vi "CPP-Multiplot.vi"(1 "Job Directory":path) -> (2 "Saved Automatically?":bool, 3 "gnuplotScript":string, 4 "Plot data file":path)   [LabVIEW 2022 SP3]
uses:
  gnuplotScriptComponents/plotstyle.ctl
  gnuplotScriptComponents/graphPeripherals.ctl
  gnuplotScriptComponents/minAndMax.ctl
  gnuplotScriptComponents/AutoManualNumber.ctl
  gnuplotScriptComponents/ticsAndGrids.ctl
  gnuplotScriptComponents/tics.ctl
  gnuplotScriptComponents/grids.ctl
  gnuplotScriptComponents/legendProperties.ctl
  gnuplotScriptComponents/legendAppearance.ctl
  gnuplotScriptComponents/alignment.ctl
  gnuplotScriptComponents/at.ctl
  gnuplotScriptComponents/margins.ctl
  gnuplotScriptComponents/source.ctl
  gnuplotScriptComponents/Master_Legend.ctl
  gnuplotScriptComponents/MasterPeripherals.ctl
  Error bar Type.ctl
  gnuplotScriptComponents/axisName.ctl
  Results_plotter_Global.vi
  Data plotting/subVIs/Plot_Values_Global.vi
panel:
  out "Multi_Plot":bool
  in  "OpenLogfile?":bool
  in  "Show Script Editor?":bool
  in  "Tab Control":T1(tab)=enum."Appearance"
  in  "setupPath":path
  in  "saveMPsetup":bool
  in  "loadMPsetup":bool
  in  "Each Graph contains:":T2=enum."Series"
  in  "Rows from:":T2=enum."Until done"
  in  "Columns from:":T2=enum."Yellow Filter"
  in  "Margins":T3={"Top"=2.0, "Bottom"=2.0, "Left"=2.0, "Right"=2.0}
  in  "Height (in)":dbl=7.0 min=0.5 step=0.5 format="%.1f"
  in  "Width (in)":dbl=10.0 min=0.5 step=0.5 format="%.1f"
  in  "nRows":u8=3 min=1
  in  "nCols":u8=3 min=1
  in  "ScaleAdjust":dbl=0.9 min=0.1 max=2.0 step=0.1
  in  "Swop Series and Plots":bool
  in  "PlotTitlesNeed $$?":bool=TRUE
  in  "Show Channels with range of Values?":bool
  in  "ManualPlotTitles":string[](array[string])
  out "AutoPlotTitles":string[](array[string])
  in  "Individual Plot Titles":bool=TRUE
  in  "Page Title Pre Block":string
  in  "Page Title Post Block":string
  in  "Values to include in Page Title":i32[](listbox)
  in  "Plot Title Offset (characters)":cluster{"horizontal":dbl, "vertical":dbl}
  out "Final Title":string
  in  "PlotNamesNeed $$?":bool=TRUE
  in  "Plot Legends Manual":string[](array[string])
  in  "Plotstyles":T4[](array[typedef])=[{"Style"="linespoints", "Color"=16711680, "PointType"=1, "PointSize"=1.0, "LineWidth"=1.0, "LineType"=1}, {"Style"="linespoints", "Color"=16860, "PointType"=2, "PointSize"=1.0, "LineWidth"=1.0, "LineType"=1}, {"Style"="linespoints", "Color"=51228, "PointType"=3, "PointSize"=1.0, "LineWidth"=1.0, "LineType"=1}, {"Style"="linespoints", "Color"=0, "PointType"=4, "PointSize"=1.0, "LineWidth"=1.0, "LineType"=1}, {"Style"="linespoints", "Color"=9567230, "PointType"=5, "PointSize"=1.0, "LineWidth"=1.0, "LineType"=1}, {"Style"="linespoints", "Color"=12369084, "PointType"=6, "PointSize"=1.0, "LineWidth"=1.0, "LineType"=1}, {"Style"="linespoints", "Color"=15667967, "PointType"=7, "PointSize"=1.0, "LineWidth"=1.0, "LineType"=1}, {"Style"="linespoints", "Color"=15400704, "PointType"=8, "PointSize"=1.0, "LineWidth"=1.0, "LineType"=1}, {"Style"="linespoints", "Color"=128, "PointType"=9, "PointSize"=1.0, "LineWidth"=1.0, "LineType"=1}, {"Style"="linespoints", "Color"=8404992, "PointType"=10, "PointSize"=1.0, "LineWidth"=1.0, "LineType"=1}, {"Style"="linespoints", "Color"=6737151, "PointType"=11, "PointSize"=1.0, "LineWidth"=1.0, "LineType"=1}, {"Style"="linespoints", "Color"=8388672, "PointType"=12, "PointSize"=1.0, "LineWidth"=1.0, "LineType"=1}, {"Style"="linespoints", "Color"=16740303, "PointType"=13, "PointSize"=1.0, "LineWidth"=1.0, "LineType"=1}, {"Style"="linespoints", "Color"=16764006, "PointType"=14, "PointSize"=1.0, "LineWidth"=1.0, "LineType"=1}, {"Style"="linespoints", "Color"=8421376, "PointType"=15, "PointSize"=1.0, "LineWidth"=1.0, "LineType"=1}, {"Style"="linespoints", "Color"=65408, "PointType"=16, "PointSize"=1.0, "LineWidth"=1.0, "LineType"=1}] caption="Style                              Colour  PointType    PointSize     Linewidth      Linestyle" {"LineType" min=1 max=6 step=1; "LineWidth" min=1 max=6 step=1; "PointSize" min=0 step=0.1}
  out "Plot Legends Auto":string[](array[string])
  out "No of Series supplied":i32
  out "No of Graph Slots Available":i32
  in  "Plot Legends":bool=TRUE
  in  "Error Bar Type":T5=enum."Standard Error"
  in  "X axis label":enum32{"Autolabel", "Manual Label"}(tab)
  out "X or theta label":string
  in  "X or theta label Manual":string
  in  "LegendProperties":T6={"Appearance"={"layout"="", "text-sample order"="", "key order"="", "surroundingBox"="", "MaxRows"=0, "MaxCols"=0, "WidthAdjust"=0.0}, "Alignment"={"Horizontal"="", "Vertical"=""}, "Location"="auto", "\"At\" location"={"XcoordSys"="", "YcoordSys"="", "Xvalue"=0.0, "Yvalue"=0.0}}
  in  "Y/R tics And Grids":T10={"tics"={"ticMin"=0.0, "ticStep"=5.0, "ticMax"=0.0, "minorDivsPerMajor"=2, "ticSpacing"=enum."Approx n Tics (rounded)", "ticPosition"=enum."Inside, no mirror"}, "Grids"={"Gridlines"=enum."No grids", "Zeroaxis"=enum."No zero axis"}, "Mapping"=enum."Lin"}
  in  "X/Theta tics And Grids":T10={"tics"={"ticMin"=0.0, "ticStep"=5.0, "ticMax"=0.0, "minorDivsPerMajor"=2, "ticSpacing"=enum."Approx n Tics (rounded)", "ticPosition"=enum."Inside, no mirror"}, "Grids"={"Gridlines"=enum."Major grid", "Zeroaxis"=enum."No zero axis"}, "Mapping"=enum."Lin"}
  in  "PlotType":enum32{"XY", "Polar", "Time"}(tab)
  in  "yAxisBounds":T13={"Min"={"Auto"=TRUE, "Value"=0.0}, "Max"={"Auto"=TRUE, "Value"=0.0}}
  in  "Additional XYgnuplot":string
  in  "xAxisBounds":T13={"Min"={"Auto"=TRUE, "Value"=0.0}, "Max"={"Auto"=TRUE, "Value"=0.0}}
  in  "Set bounds using XY Plot \non Results file plotter":bool
  in  "Angle Units":bool=TRUE
  in  "AngleMode":string(combo)="Compass"
  in  "wrapGapsUpTo:":dbl=30.0 step=0.1
  in  "Additional Polar gnuplot":string
  in  "rAxisBounds":T13={"Min"={"Auto"=FALSE, "Value"=0.0}, "Max"={"Auto"=FALSE, "Value"=1.5}}
  out "Time format?":bool
  in  "Time/Date Format":string(combo)="%I:%M %p\\n%d-%b-%y"
  in  "Select Time Zone":u32(ring)=142 items=["Abbreviation (Time Zone Name)", "A (Alpha Time Zone)", "ACDT (Australian Central Daylight Time  CDT ÇƒÏ Central Daylight Time CDST ÇƒÏ Central Daylight Savings Time)", "ACST (Australian Central Standard Time  CST ÇƒÏ Central Standard Time)", "ACT (Acre Time)", "ACT (Australian Central Time)", "ACWST (Australian Central Western Standard Time)", "ADT (Arabia Daylight Time  AST ÇƒÏ Arabia Summer Time)", "ADT (Atlantic Daylight Time  ADST ÇƒÏ Atlantic Daylight Saving Time AST ÇƒÏ Atlantic Summer Time  HAA ÇƒÏ Heure Avancv©e de l'Atlantique (French))", "AEDT (Australian Eastern Daylight Time  EDT ÇƒÏ Eastern Daylight Time EDST ÇƒÏ Eastern Daylight Saving Time)", "AEST (Australian Eastern Standard Time  EST ÇƒÏ Eastern Standard Time AET ÇƒÏ Australian Eastern Time)", "AET (Australian Eastern Time)", "AFT (Afghanistan Time)", "AKDT (Alaska Daylight Time  ADST ÇƒÏ Alaska Daylight Saving Time)", "AKST (Alaska Standard Time  AT ÇƒÏ Alaska Time)", "ALMT (Alma-Ata Time)", "AMST (Amazon Summer Time)", "AMST (Armenia Summer Time  AMDT ÇƒÏ Armenia Daylight Time)", "AMT (Amazon Time)", "AMT (Armenia Time)", "ANAST (Anadyr Summer Time)", "ANAT (Anadyr Time)", "AQTT (Aqtobe Time)", "ART (Argentina Time)", "AST (Arabia Standard Time  AST ÇƒÏ Arabic Standard Time AST ÇƒÏ Al Manamah Standard Time)", "AST (Atlantic Standard Time  AT ÇƒÏ Atlantic Time  AST ÇƒÏ Tiempo Estv∞ndar del Atlv∞ntico (Spanish) HNA ÇƒÏ Heure Normale de l'Atlantique (French))", "AT (Atlantic Time)", "AWDT (Australian Western Daylight Time  WDT ÇƒÏ Western Daylight Time WST ÇƒÏ Western Summer Time)", "AWST (Australian Western Standard Time  WST ÇƒÏ Western Standard Time WAT ÇƒÏ Western Australia Time)", "AZOST (Azores Summer Time  AZODT ÇƒÏ Azores Daylight Time)", "AZOT (Azores Time  AZOST ÇƒÏ Azores Standard Time)", "AZST (Azerbaijan Summer Time)", "AZT (Azerbaijan Time)", "AoE (Anywhere on Earth)", "B (Bravo Time Zone)", "BNT (Brunei Darussalam Time  BDT ÇƒÏ Brunei Time)", "BOT (Bolivia Time)", "BRST (Brasv?lia Summer Time  BST ÇƒÏ Brazil Summer Time BST ÇƒÏ Brazilian Summer Time)", "BRT (Brasv?lia Time  BT ÇƒÏ Brazil Time BT ÇƒÏ Brazilian Time)", "BST (Bangladesh Standard Time)", "BST (Bougainville Standard Time)", "BST (British Summer Time  BDT ÇƒÏ British Daylight Time BDST ÇƒÏ British Daylight Saving Time)", "BTT (Bhutan Time)", "C (Charlie Time Zone)", "CAST (Casey Time)", "CAT (Central Africa Time)", "CCT (Cocos Islands Time)", "CDT (Central Daylight Time  CDST ÇƒÏ Central Daylight Saving Time NACDT ÇƒÏ North American Central Daylight Time  HAC ÇƒÏ Heure Avancv©e du Centre (French))", "CDT (Cuba Daylight Time)", "CEST (Central European Summer Time  CEDT ÇƒÏ Central European Daylight Time ECST ÇƒÏ European Central Summer Time  MESZ ÇƒÏ Mitteleuropvßische Sommerzeit (German))", "CET (Central European Time  ECT ÇƒÏ European Central Time CET ÇƒÏ Central Europe Time  MEZ ÇƒÏ Mitteleuropvßische Zeit (German))", "CHADT (Chatham Island Daylight Time  CDT ÇƒÏ Chatham Daylight Time)", "CHAST (Chatham Island Standard Time)", "CHOST (Choibalsan Summer Time  CHODT ÇƒÏ Choibalsan Daylight Time CHODST ÇƒÏ Choibalsan Daylight Saving Time)", "CHOST (Choibalsan Summer Time)", "CHOT (Choibalsan Time)", "CHUT (Chuuk Time)", "CIDST (Cayman Islands Daylight Saving Time)", "CIST (Cayman Islands Standard Time  CIT ÇƒÏ Cayman Islands Time)", "CKT (Cook Island Time)", "CLST (Chile Summer Time  CLDT ÇƒÏ Chile Daylight Time)", "CLT (Chile Standard Time  CT ÇƒÏ Chile Time CLST ÇƒÏ Chile Standard Time)", "COT (Colombia Time)", "CST (Central Standard Time  CT ÇƒÏ Central Time NACST ÇƒÏ North American Central Standard Time  CST ÇƒÏ Tiempo Central Estv∞ndar (Spanish) HNC ÇƒÏ Heure Normale du Centre (French))", "CST (China Standard Time)", "CST (Cuba Standard Time)", "CT (Central Time)", "CVT (Cape Verde Time)", "CXT (Christmas Island Time)", "ChST (Chamorro Standard Time  GST ÇƒÏ Guam Standard Time)", "D (Delta Time Zone)", "DAVT (Davis Time)", "DDUT (Dumont-d'Urville Time)", "E (Echo Time Zone)", "EASST (Easter Island Summer Time  EADT ÇƒÏ Easter Island Daylight Time)", "EAST (Easter Island Standard Time)", "EAT (Eastern Africa Time  EAT ÇƒÏ East Africa Time)", "ECT (Ecuador Time)", "EDT (Eastern Daylight Time  EDST ÇƒÏ Eastern Daylight Savings Time NAEDT ÇƒÏ North American Eastern Daylight Time  HAE ÇƒÏ Heure Avancv©e de l'Est (French) EDT ÇƒÏ Tiempo de verano del Este (Spanish))", "EEST (Eastern European Summer Time  EEDT ÇƒÏ Eastern European Daylight Time  OESZ ÇƒÏ Osteuropvßische Sommerzeit (German))", "EET (Eastern European Time  OEZ ÇƒÏ Osteuropvßische Zeit (German))", "EGST (Eastern Greenland Summer Time  EGST ÇƒÏ East Greenland Summer Time)", "EGT (East Greenland Time  EGT ÇƒÏ Eastern Greenland Time)", "EST (Eastern Standard Time  ET ÇƒÏ Eastern Time  NAEST ÇƒÏ North American Eastern Standard Time  ET ÇƒÏ Tiempo del Este (Spanish) HNE ÇƒÏ Heure Normale de l'Est (French))", "ET (Eastern Time)", "F (Foxtrot Time Zone)", "FET (Further-Eastern European Time)", "FJST (Fiji Summer Time  FJDT ÇƒÏ Fiji Daylight Time)", "FJT (Fiji Time)", "FKST (Falkland Islands Summer Time  FKDT ÇƒÏ Falkland Island Daylight Time)", "FKT (Falkland Island Time  FKST ÇƒÏ Falkland Island Standard Time)", "FNT (Fernando de Noronha Time)", "G (Golf Time Zone)", "GALT (Galapagos Time)", "GAMT (Gambier Time  GAMT ÇƒÏ Gambier Islands Time)", "GET (Georgia Standard Time)", "GFT (French Guiana Time)", "GILT (Gilbert Island Time)", "GMT (Greenwich Mean Time  \"ÇƒÏ Coordinated Universal Time GT ÇƒÏ Greenwich Time)", "GST (Gulf Standard Time)", "GST (South Georgia Time)", "GYT (Guyana Time)", "H (Hotel Time Zone)", "HADT (Hawaii-Aleutian Daylight Time  HDT ÇƒÏ Hawaii Daylight Time)", "HAST (Hawaii-Aleutian Standard Time  HST ÇƒÏ Hawaii Standard Time)", "HKT (Hong Kong Time)", "HOVST (Hovd Summer Time  HOVDT ÇƒÏ Hovd Daylight Time HOVDST ÇƒÏ Hovd Daylight Saving Time)", "HOVST (Hovd Summer Time)", "HOVT (Hovd Time)", "I (India Time Zone)", "ICT (Indochina Time)", "IDT (Israel Daylight Time)", "IOT (Indian Chagos Time)", "IRDT (Iran Daylight Time  IRST ÇƒÏ Iran Summer Time IDT ÇƒÏ Iran Daylight Time)", "IRKST (Irkutsk Summer Time)", "IRKT (Irkutsk Time)", "IRST (Iran Standard Time  IT ÇƒÏ Iran Time)", "IST (India Standard Time  IT ÇƒÏ India Time IST ÇƒÏ Indian Standard Time)", "IST (Irish Standard Time  IST ÇƒÏ Irish Summer Time)", "IST (Israel Standard Time)", "JST (Japan Standard Time)", "K (Kilo Time Zone)", "KGT (Kyrgyzstan Time)", "KOST (Kosrae Time)", "KRAST (Krasnoyarsk Summer Time)", "KRAT (Krasnoyarsk Time)", "KST (Korea Standard Time  KST ÇƒÏ Korean Standard Time KT ÇƒÏ Korea Time)", "KUYT (Kuybyshev Time  SAMST ÇƒÏ Samara Summer Time)", "L (Lima Time Zone)", "LHDT (Lord Howe Daylight Time)", "LHST (Lord Howe Standard Time)", "LINT (Line Islands Time)", "M (Mike Time Zone)", "MAGST (Magadan Summer Time  MAGST ÇƒÏ Magadan Island Summer Time)", "MAGT (Magadan Time  MAGT ÇƒÏ Magadan Island Time)", "MART (Marquesas Time)", "MAWT (Mawson Time)", "MDT (Mountain Daylight Time  MDST ÇƒÏ Mountain Daylight Saving Time NAMDT ÇƒÏ North American Mountain Daylight Time  HAR ÇƒÏ Heure Avancv©e des Rocheuses (French))", "MHT (Marshall Islands Time)", "MMT (Myanmar Time)", "MSD (Moscow Daylight Time  Moscow Summer Time)", "MSK (Moscow Standard Time  MCK ÇƒÏ Moscow Time)", "MST (Mountain Standard Time  MT ÇƒÏ Mountain Time NAMST ÇƒÏ North American Mountain Standard Time  HNR ÇƒÏ Heure Normale des Rocheuses (French))", "MT (Mountain Time)", "MUT (Mauritius Time)", "MVT (Maldives Time)", "MYT (Malaysia Time  MST ÇƒÏ Malaysian Standard Time)", "N (November Time Zone)", "NCT (New Caledonia Time)", "NDT (Newfoundland Daylight Time  HAT ÇƒÏ Heure Avancv©e de Terre-Neuve (French))", "NFT (Norfolk Time  NFT ÇƒÏ Norfolk Island Time)", "NOVST (Novosibirsk Summer Time  OMSST ÇƒÏ Omsk Summer Time)", "NOVT (Novosibirsk Time  OMST ÇƒÏ Omsk Standard Time)", "NPT (Nepal Time)", "NRT (Nauru Time)", "NST (Newfoundland Standard Time  HNT ÇƒÏ Heure Normale de Terre-Neuve (French))", "NUT (Niue Time)", "NZDT (New Zealand Daylight Time)", "NZST (New Zealand Standard Time)", "O (Oscar Time Zone)", "OMSST (Omsk Summer Time  NOVST ÇƒÏ Novosibirsk Summer Time)", "OMST (Omsk Standard Time  OMST ÇƒÏ Omsk Time NOVT ÇƒÏ Novosibirsk Time)", "ORAT (Oral Time)", "P (Papa Time Zone)", "PDT (Pacific Daylight Time  PDST ÇƒÏ Pacific Daylight Saving Time NAPDT ÇƒÏ North American Pacific Daylight Time  HAP ÇƒÏ Heure Avancv©e du Pacifique (French))", "PET (Peru Time)", "PETST (Kamchatka Summer Time)", "PETT (Kamchatka Time  PETT ÇƒÏ Petropavlovsk-Kamchatski Time)", "PGT (Papua New Guinea Time)", "PHOT (Phoenix Island Time)", "PHT (Philippine Time  PST ÇƒÏ Philippine Standard Time)", "PKT (Pakistan Standard Time  PKT ÇƒÏ Pakistan Time)", "PMDT (Pierre & Miquelon Daylight Time)", "PMST (Pierre & Miquelon Standard Time)", "PONT (Pohnpei Standard Time)", "PST (Pacific Standard Time  PT ÇƒÏ Pacific Time NAPST ÇƒÏ North American Pacific Standard Time  PT ÇƒÏ Tiempo del Pacv?fico (Spanish) HNP ÇƒÏ Heure Normale du Pacifique (French))", "PST (Pitcairn Standard Time)", "PT (Pacific Time)", "PWT (Palau Time)", "PYST (Paraguay Summer Time)", "PYT (Paraguay Time)", "PYT (Pyongyang Time  PYST ÇƒÏ Pyongyang Standard Time)", "PYT (Pyongyang Time)", "Q (Quebec Time Zone)", "QYZT (Qyzylorda Time)", "R (Romeo Time Zone)", "RET (Reunion Time)", "ROTT (Rothera Time)", "S (Sierra Time Zone)", "SAKT (Sakhalin Time)", "SAMT (Samara Time  SAMT ÇƒÏ Samara Standard Time)", "SAST (South Africa Standard Time  SAST ÇƒÏ South African Standard Time)", "SBT (Solomon Islands Time  SBT ÇƒÏ Solomon Island Time)", "SCT (Seychelles Time)", "SGT (Singapore Time  SST ÇƒÏ Singapore Standard Time)", "SRET (Srednekolymsk Time)", "SRT (Suriname Time)", "SST (Samoa Standard Time)", "SYOT (Syowa Time)", "T (Tango Time Zone)", "TAHT (Tahiti Time)", "TFT (French Southern and Antarctic Time  KIT ÇƒÏ Kerguelen (Islands) Time)", "TJT (Tajikistan Time)", "TKT (Tokelau Time)", "TLT (East Timor Time)", "TMT (Turkmenistan Time)", "TOT (Tonga Time)", "TVT (Tuvalu Time)", "U (Uniform Time Zone)", "ULAST (Ulaanbaatar Summer Time  ULAST ÇƒÏ Ulan Bator Summer Time)", "ULAST (Ulaanbaatar Summer Time)", "ULAT (Ulaanbaatar Time  ULAT ÇƒÏ Ulan Bator Time)", "ULAT (Ulaanbaatar Time)", "UTC (Coordinated Universal Time)", "UYST (Uruguay Summer Time)", "UYT (Uruguay Time)", "UZT (Uzbekistan Time)", "V (Victor Time Zone)", "VET (Venezuelan Standard Time  HLV ÇƒÏ Hora Legal de Venezuela (Spanish))", "VLAST (Vladivostok Summer Time)", "VLAT (Vladivostok Time)", "VOST (Vostok Time)", "VUT (Vanuatu Time  EFATE ÇƒÏ Efate Time)", "W (Whiskey Time Zone)", "WAKT (Wake Time)", "WARST (Western Argentine Summer Time)", "WAST (West Africa Summer Time)", "WAT (West Africa Time)", "WEST (Western European Summer Time  WEDT ÇƒÏ Western European Daylight Time  WESZ ÇƒÏ Westeuropvßische Sommerzeit (German))", "WET (Western European Time  GMT ÇƒÏ Greenwich Mean Time  WEZ ÇƒÏ Westeuropvßische Zeit (German))", "WFT (Wallis and Futuna Time)", "WGST (Western Greenland Summer Time  WGST ÇƒÏ West Greenland Summer Time)", "WGT (West Greenland Time  WGT ÇƒÏ Western Greenland Time)", "WIB (Western Indonesian Time  WIB ÇƒÏ Waktu Indonesia Barat)", "WIT (Eastern Indonesian Time  WIT ÇƒÏ Waktu Indonesia Timur)", "WITA (Central Indonesian Time  WITA ÇƒÏ Waktu Indonesia Tengah)", "WST (West Samoa Time  ST ÇƒÏ Samoa Time)", "WST (Western Sahara Summer Time)", "WT (Western Sahara Standard Time  WT ÇƒÏ Western Sahara Time)", "X (X-ray Time Zone)", "Y (Yankee Time Zone)", "YAKST (Yakutsk Summer Time)", "YAKT (Yakutsk Time)", "YAPT (Yap Time)", "YEKST (Yekaterinburg Summer Time)", "YEKT (Yekaterinburg Time)", "Z (Zulu Time Zone)"]
  out "Time Format String":string="%I:%M %p\\n%d-%b-%y"
  out "Formatted date/time string":string="05:00 PM\\n21-Jan-16"
  out "TZ Shift (hrs)":string="UTC-7.00"
  in  "Y axis label":enum32{"Autolabel", "Manual Label"}(tab)
  out "Y or R label":string
  in  "Y or R label Manual 2":string
  in  "PeripheralsMasterControl":T15=enum."Edges Only"
  in  "Legend Options":T16=enum."Single Legend Below table"
  in  "GraphPeripherals":T17[][](array[typedef])
  out "PlotCommand":string
  in  "Filename Max length":i32=55
  out "File Path Control":path
  out "AuditTrail":string[](array[string])
  out "Desired Legends":string[][](array[string])
  out "original name had conflict":bool
  out "crossplatform problem":bool
  # "Rows/ Columns/ Series from: controls not wired- just a thought for explicit control of what goes where...?"
  # "Overall Page Title"
  # "There are as many graphs as there are titles (from Selector 2)...."
  # "Plot Styles"
  # "Each graph contains plots from Selector 1..."
  # "X/theta"
  # "Y/r"
  # "Shows the numbered line colours and point styles available- well it would, if it didn't disappear every time I update from the repository..!"
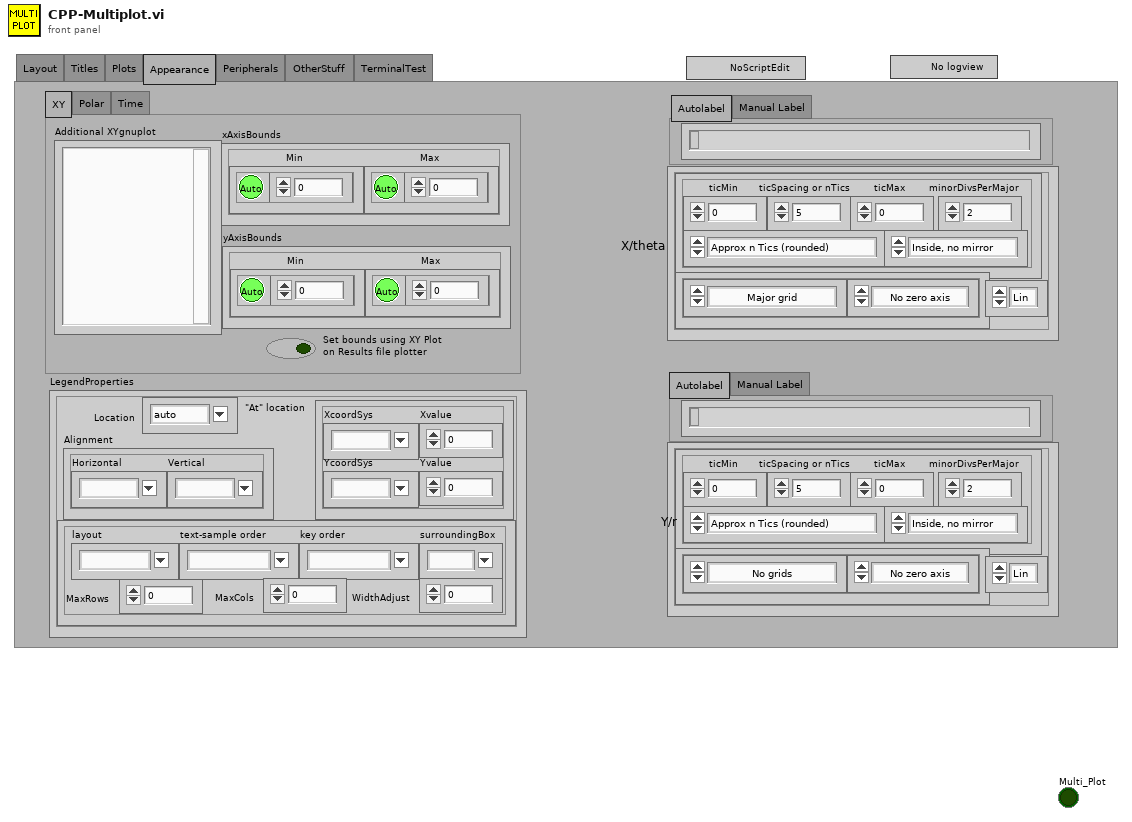
[diagram p1: front panel]
types:
  T1 = enum32{"Layout", "Titles", "Plots", "Appearance", "Peripherals", "OtherStuff ", "TerminalTest"}
  T2 = typedef "source.ctl" = enum16{"Specified:", "Yellow Filter", "Red Filter", "Until done", "Series"}
  T3 = typedef "margins.ctl" = cluster{"Top":dbl, "Bottom":dbl, "Left":dbl, "Right":dbl}
  T4 = typedef "plotstyle.ctl" = cluster{"Style":string, "Color":u32, "PointType":i32, "PointSize":sgl, "LineWidth":sgl, "LineType":u8}
  T5 = typedef "Error bar Type.ctl" = enum16{"None", "Standard Error", "Separate upper and lower"}
  T6 = typedef "legendProperties.ctl" = cluster{"Appearance":T7, "Alignment":T8, "Location":string, "\"At\" location":T9}
  T7 = typedef "legendAppearance.ctl" = cluster{"layout":string, "text-sample order":string, "key order":string, "surroundingBox":string, "MaxRows":u32, "MaxCols":u32, "WidthAdjust":dbl}
  T8 = typedef "alignment.ctl" = cluster{"Horizontal":string, "Vertical":string}
  T9 = typedef "at.ctl" = cluster{"XcoordSys":string, "YcoordSys":string, "Xvalue":dbl, "Yvalue":dbl}
  T10 = typedef "ticsAndGrids.ctl" = cluster{"tics":T11, "Grids":T12, "Mapping":enum8{"Lin", "Log"}}
  T11 = typedef "tics.ctl" = cluster{"ticMin":dbl, "ticStep":dbl, "ticMax":dbl, "minorDivsPerMajor":i32, "ticSpacing":enum16{"Auto Tics", "Fixed spacing", "Fixed Minimum and Spacing", "Start, Spacing and Maximum", "Approx n Tics (rounded)"}, "ticPosition":enum16{"Inside, no mirror", "Inside, mirrored", "Outside, no mirror", "Outside, mirrored", "Invisible"}}
  T12 = typedef "grids.ctl" = cluster{"Gridlines":enum16{"No grids", "Major grid", "Minor grid", "Major and Minor"}, "Zeroaxis":enum16{"No zero axis", "Show zero axis"}}
  T13 = typedef "minAndMax.ctl" = cluster{"Min":T14, "Max":T14}
  T14 = typedef "AutoManualNumber.ctl" = cluster{"Auto":bool, "Value":dbl}
  T15 = typedef "MasterPeripherals.ctl" = enum16{"Use Table", "Titles On", "Edges Only", "All Off"}
  T16 = typedef "Master_Legend.ctl" = enum16{"No Legend", "Single Legend Below table", "Legend as per array"}
  T17 = typedef "graphPeripherals.ctl" = cluster{"title":bool, "key":bool, "Xtic":bool, "Ytic":bool, "Xlab":bool, "Ylab":bool}
  T18 = typedef "Error_bars.ctl" = cluster{"Upper":string[], "Lower":string[], "St Error":string[]}
  T19 = typedef "axisName.ctl" = string
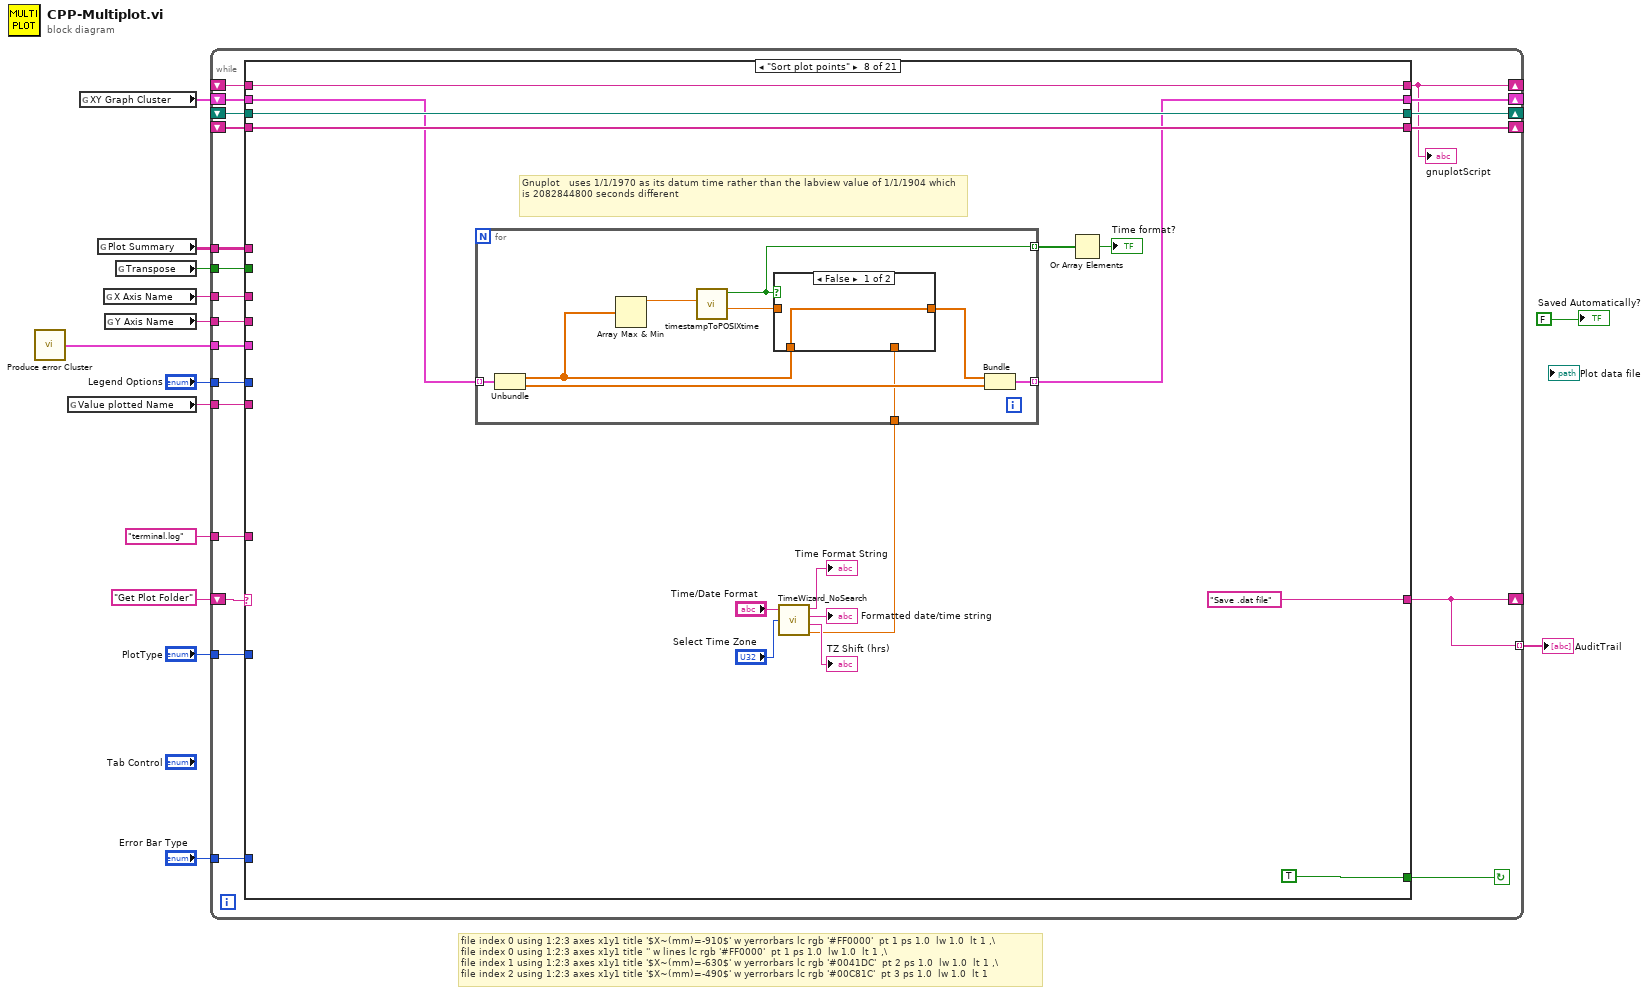
[diagram p0: block diagram]
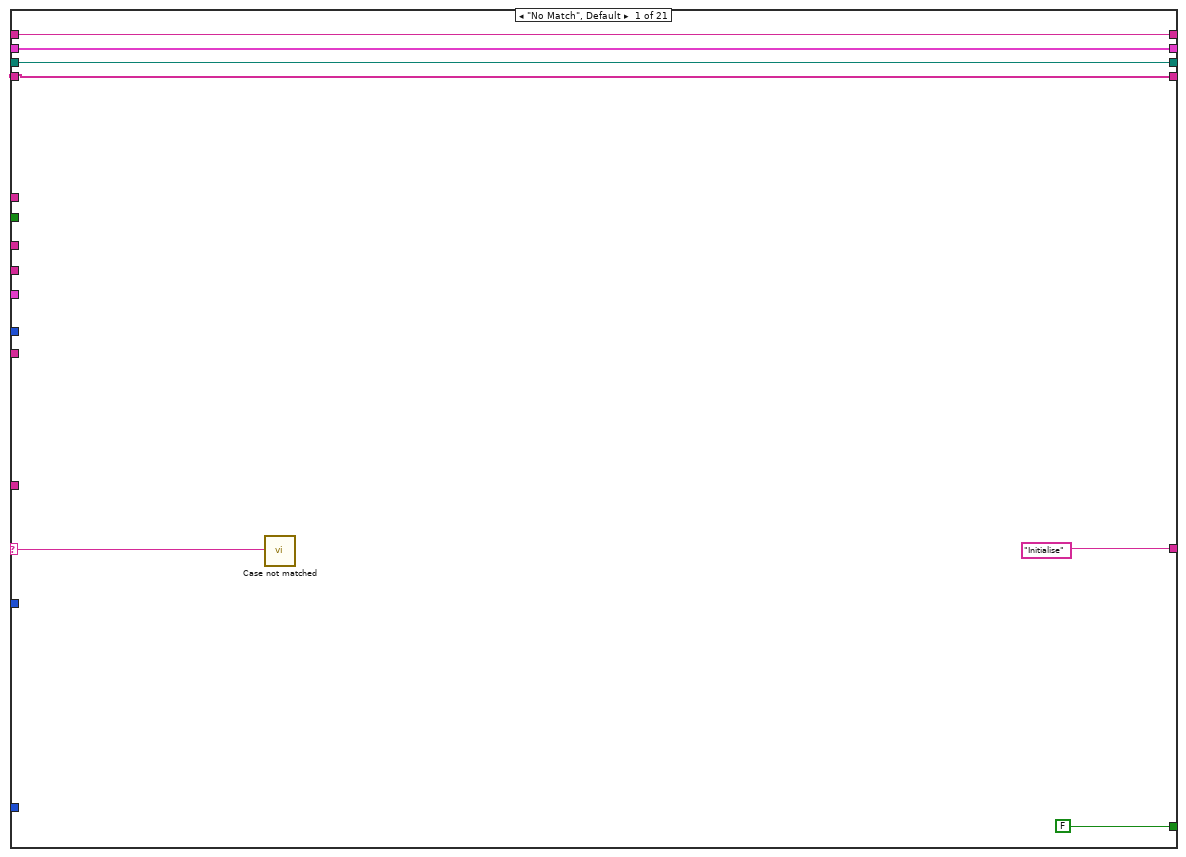
[diagram p2: hidden frame]
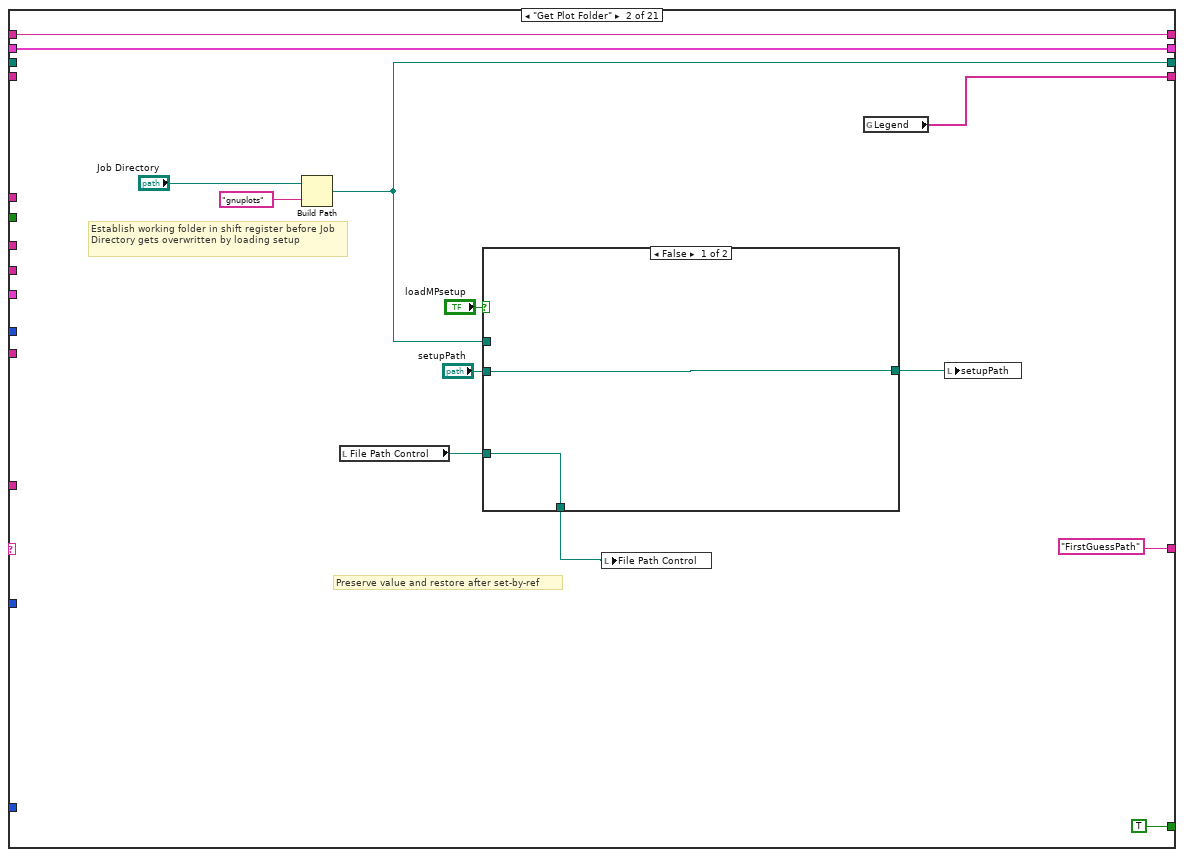
[diagram p3: hidden frame]
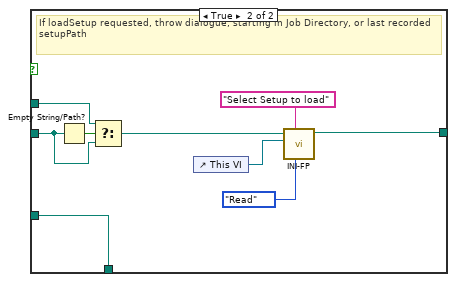
[diagram p4: hidden frame]
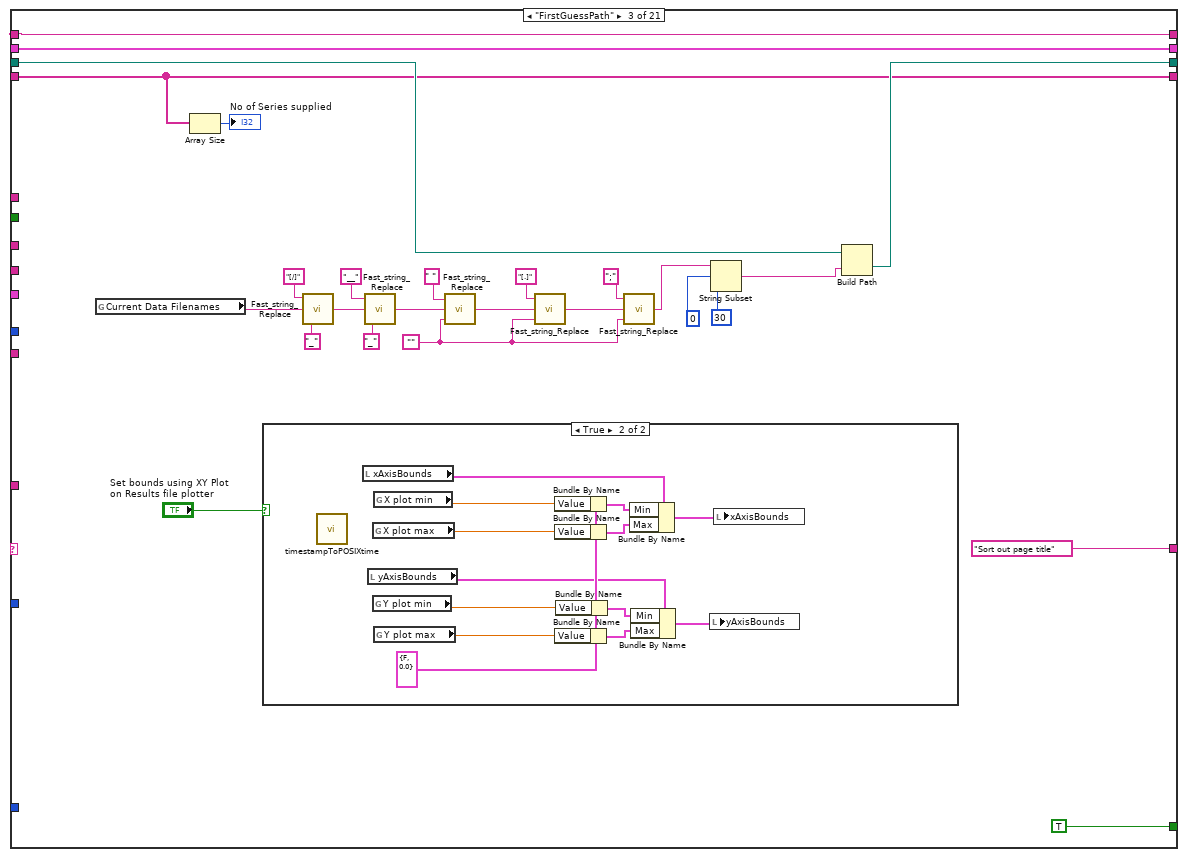
[diagram p5: hidden frame]
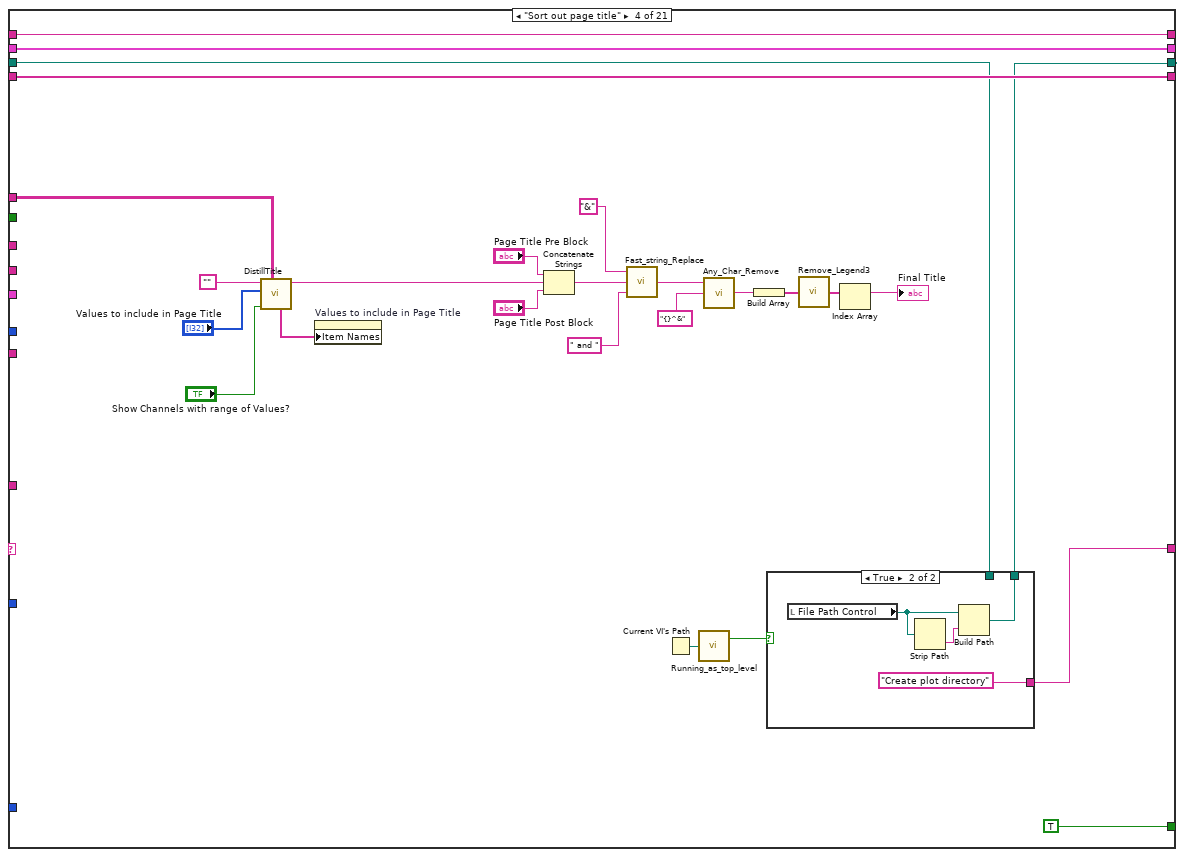
[diagram p7: hidden frame]
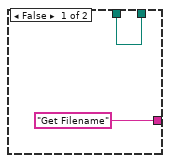
[diagram p8: hidden frame]
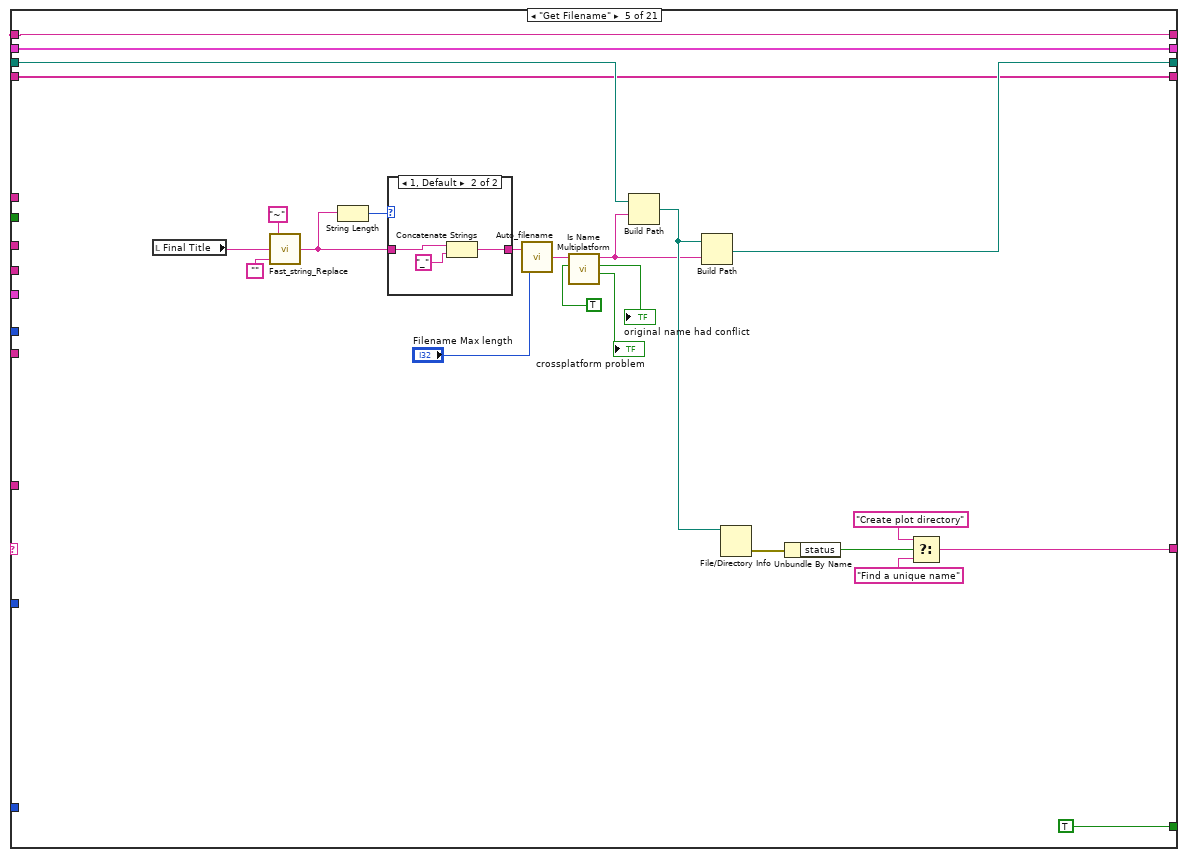
[diagram p9: hidden frame]
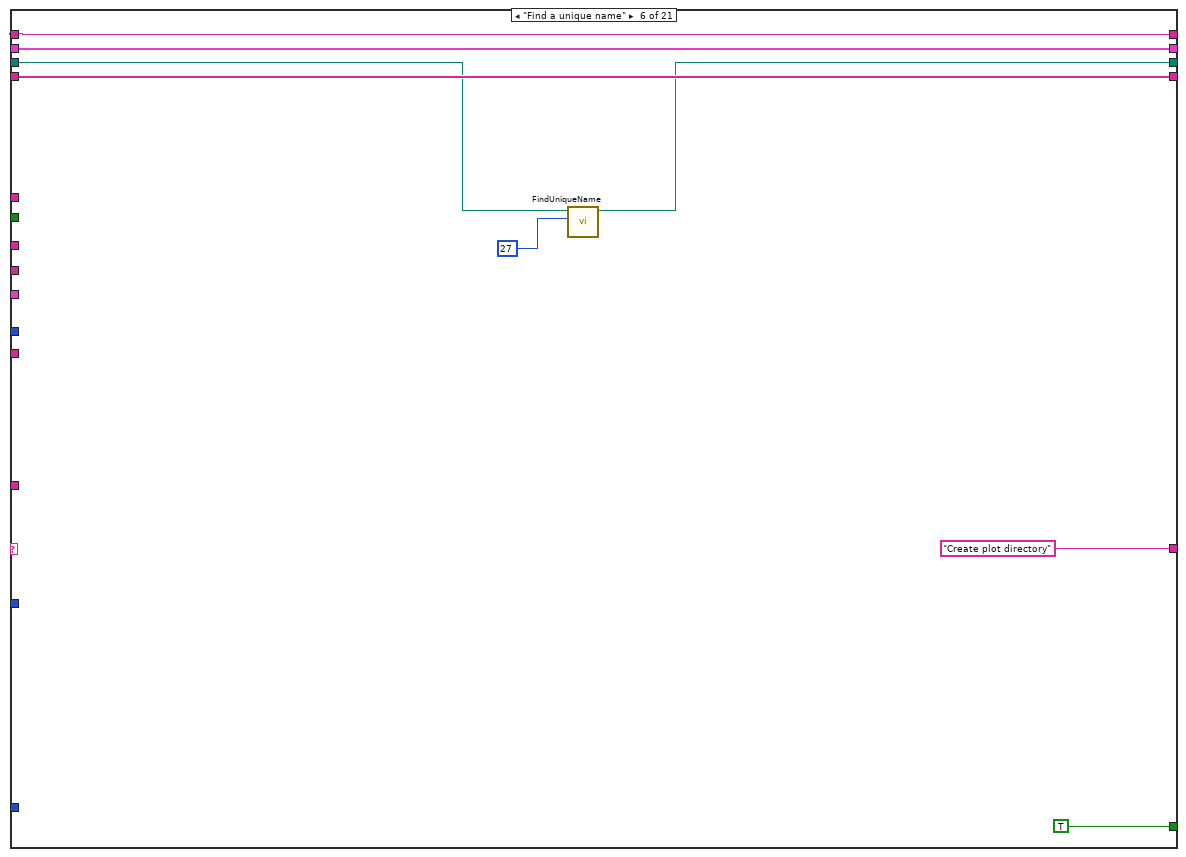
[diagram p11: hidden frame]
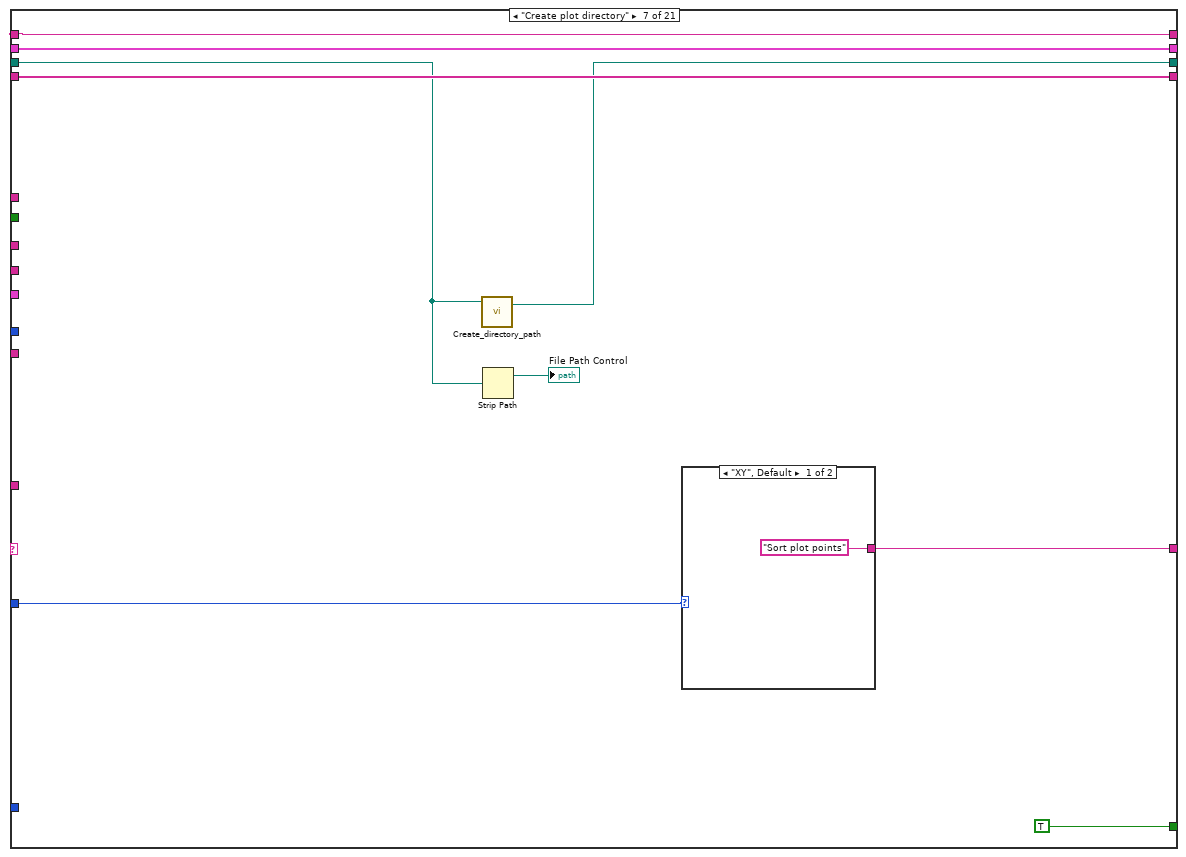
[diagram p12: hidden frame]
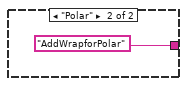
[diagram p13: hidden frame]
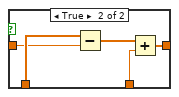
[diagram p14: hidden frame]
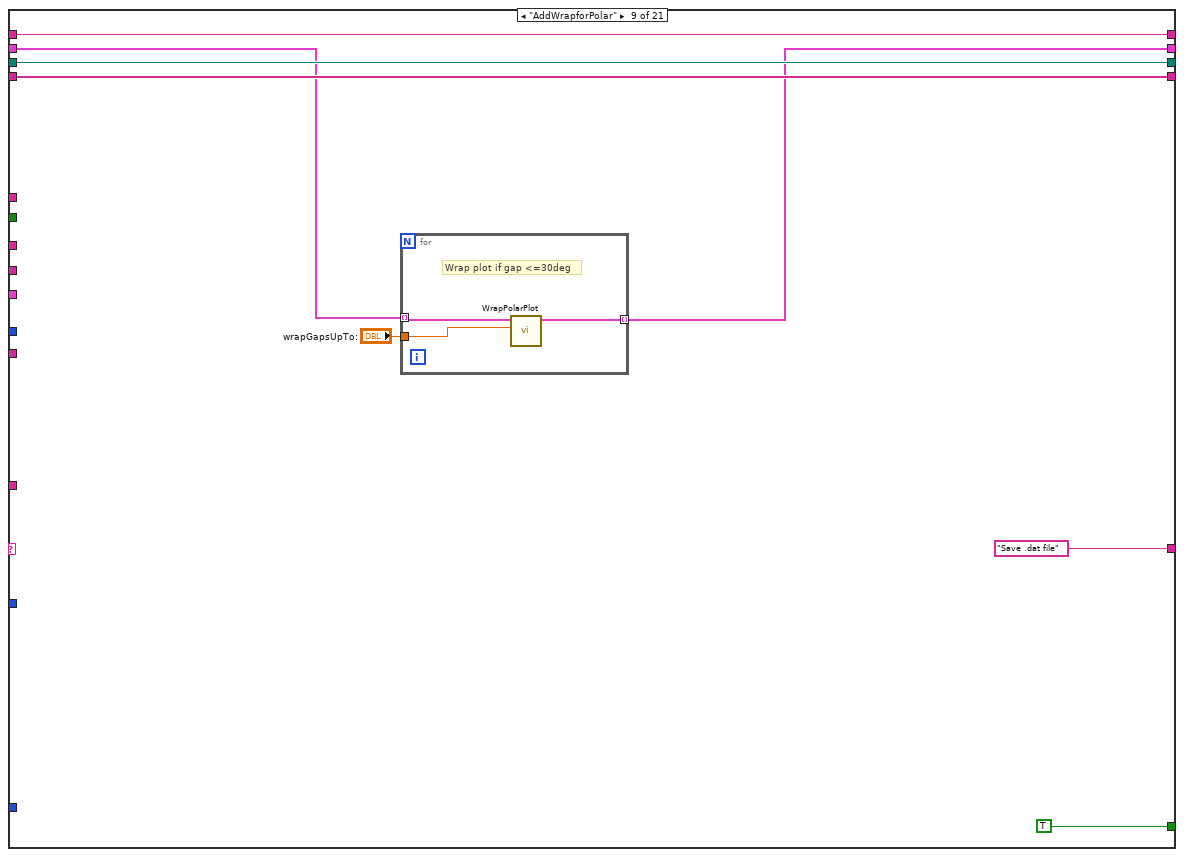
[diagram p15: hidden frame]
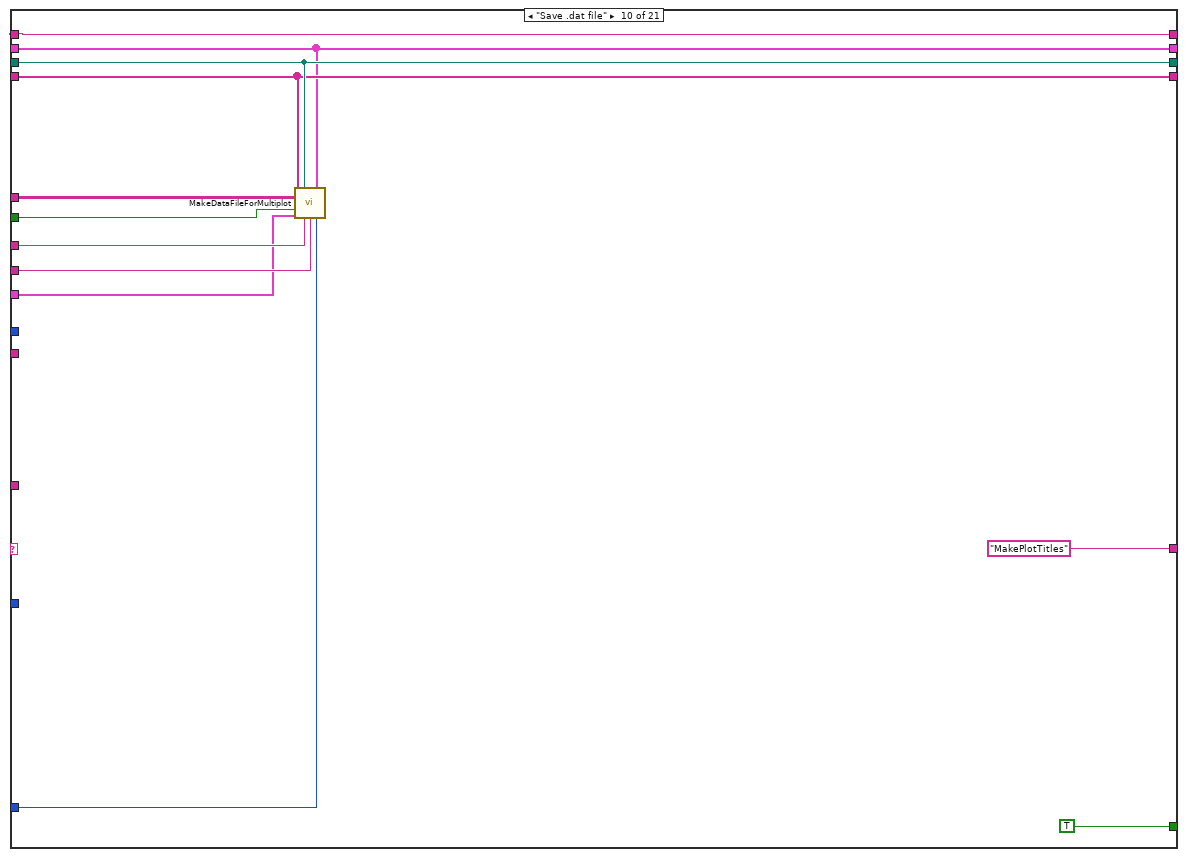
[diagram p16: hidden frame]
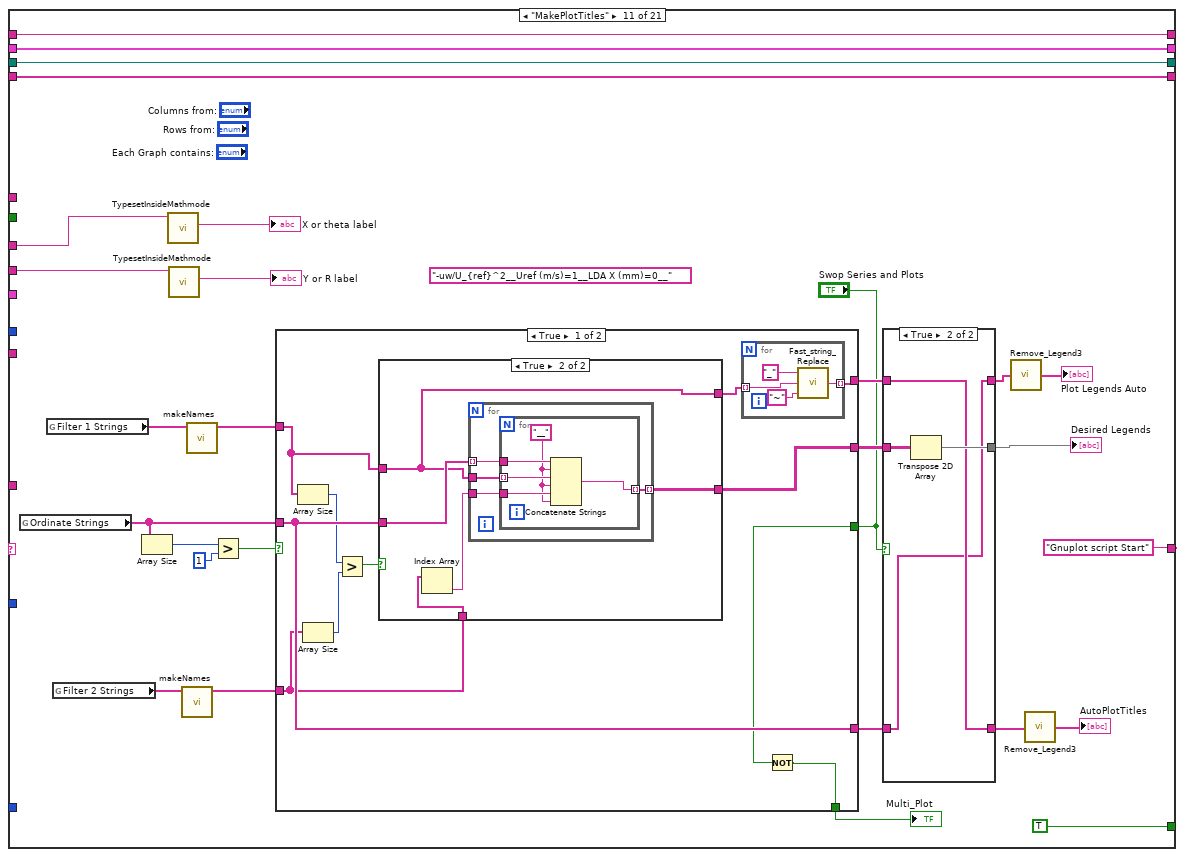
[diagram p17: hidden frame]
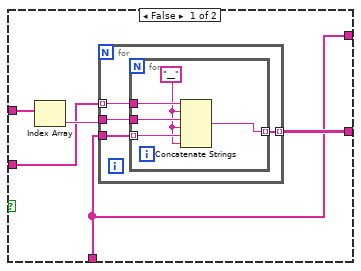
[diagram p19: hidden frame]
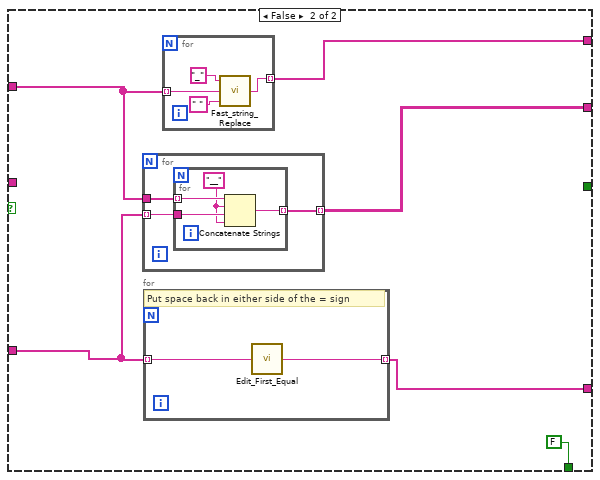
[diagram p20: hidden frame]
diagram:
  # "file index 0 using 1:2:3 axes x1y1 title '$X~(mm)=-910$' w yerrorbars lc rgb '#FF0000'  pt 1 ps 1.0  lw 1.0  lt 1 ,\\\nfile index 0 using 1:2:3 axes x1y1 title '' w lines lc rgb '#FF0000'  pt 1 ps 1.0  lw 1.0  lt 1 ,\\\nfile index 1 using 1:2:3 axes x1y1 title '$X~(mm)=-630$' w yerrorbars lc rgb '#0041DC'  pt 2 ps 1.0  lw 1.0  lt 1 ,\\\nfile index 2 using 1:2:3 axes x1y1 title '$X~(mm)=-490$' w yerrorbars lc rgb '#00C81C'  pt 3 ps 1.0  lw 1.0  lt 1"
  n1 = call "Produce error Cluster.vi"() -> ("Error Bar Cluster"=w2:T18[])  [unwired: 1 in]
  n2 = global read "Results_plotter_Global.vi" "Value plotted Name"() -> (w10:string)
  n3 = global read "Plot_Values_Global.vi" "XY Graph Cluster"() -> (w1:cluster{dbl[], dbl[]}[])
  n4 = global read "Results_plotter_Global.vi" "Plot Summary"() -> (w13:string[][])
  n5 = global read "Results_plotter_Global.vi" "X Axis Name"() -> (w12:string)
  n6 = global read "Results_plotter_Global.vi" "Y Axis Name"() -> (w11:string)
  n7 = global read "Results_plotter_Global.vi" "Transpose"() -> (w7:bool)
  n8 = while {
    shift-left: "Get Plot Folder" -> [w34]
    shift-right: [w19] -> _
    tunnel: w13 -> [w33]
    shift-right: [w32] -> _
    shift-left: _ -> [w31]
    tunnel: w12 -> [w30]
    tunnel: w11 -> [w29]
    tunnel: w10 -> [w28]
    shift-right: [w26] -> _
    shift-left: w1 -> [w27]
    shift-right: [w20] -> _
    shift-left: _ -> [w25]
    shift-right: [w24] -> _
    shift-left: _ -> [w23]
    tunnel: "terminal.log" -> [w22]
    tunnel: w7 -> [w21]
    tunnel: [w19] -> w6 mode=indexing
    tunnel: "PlotType" -> [w18]
    tunnel: "Legend Options" -> [w17]
    tunnel: w2 -> [w16]
    tunnel: "Error Bar Type" -> [w15]
    stop <- w35 continue-if-true
    n9 = case shown="\"Sort plot points\"" w34 {
      selector: w34 -> [w36 _ _ _ _ _ _ _ _ _ _ _ _ _ _ _ _ _ _ _ _]
      tunnel: [FALSE TRUE TRUE ("Top Level") TRUE ("Top Level") TRUE ("Top Level") TRUE ("Top Level") TRUE TRUE TRUE ("Top Level") TRUE ("Top Level") TRUE ("Top Level") TRUE ("Top Level") TRUE ("Top Level") TRUE ("Top Level") TRUE ("Top Level") TRUE ("Top Level") TRUE ("Top Level") TRUE ("Top Level") FALSE ("Top Level") TRUE ("Top Level") FALSE ("Top Level")] -> w35
      tunnel: ["Initialise" "FirstGuessPath" "Sort out page title" w123 w159 "Create plot directory" w174 "Save .dat file" "Save .dat file" "MakePlotTitles" "Gnuplot script Start" w358 "Build Plot Commands" "Build Plot Commands" "Write gnuplot file" ("t") "Execute shell script" ("t") "Has pdf been generated?" ("t") w624 "End" "End" ("t") "End" ("t")] -> w19
      tunnel: w33 -> [_ _ _ w118 _ _ _ _ _ w235 _ _ _ _ _ _ _ _ _ _ _]
      tunnel: [w40 w45 w92 w125 w160 w166 w179 w199 w221 w236 w265 w349 w374 w400 w455 w603 w611 w619 w632 w642 w648] -> w32
      tunnel: w31 -> [w40 _ w89 w124 w156 w167 w178 w199 w221 w236 w265 w349 w374 w400 w455 w603 w611 w619 w632 w642 w648]
      tunnel: w30 -> [_ _ _ _ _ _ _ _ _ w234 w259 _ _ _ _ _ _ _ _ _ _]
      tunnel: w29 -> [_ _ _ _ _ _ _ _ _ w233 w258 _ _ _ _ _ _ _ _ _ _]
      tunnel: w28 -> [_ _ _ _ _ _ _ _ _ _ _ _ _ _ _ _ _ _ _ _ _]
      tunnel: w27 -> [w39 w52 w91 w131 w158 w170 w182 w194 w217 w230 w264 w361 w373 w401 w413 w609 w616 w630 w637 w647 w660]
      tunnel: [w39 w52 w91 w131 w158 w170 w182 w193 w216 w230 w264 w361 w373 w401 w413 w609 w616 w630 w637 w647 w660] -> w26
      tunnel: w25 -> [w38 w53 w90 w129 w157 w169 w181 w198 w222 w237 w263 _ w367 w395 w447 w599 w614 w628 w635 w645 w659]
      tunnel: [w38 w53 w90 w129 w157 w169 w181 w198 w222 w237 w263 w335 w369 w396 w453 w599 w614 w628 w635 w645 w659] -> w20
      tunnel: [w37 w51 w67 w130 w155 w168 w180 w197 w220 w232 w262 w360 w372 w399 w454 w604 w615 w629 w636 w646 w658] -> w24
      tunnel: w23 -> [w37 _ w67 w130 w155 w168 w180 w197 w220 w232 w262 w360 w372 w399 w454 w604 w615 w629 w636 w646 w658]
      tunnel: w22 -> [_ _ _ _ _ _ _ _ _ _ _ _ _ _ _ _ w610 _ _ w640 _]
      tunnel: w21 -> [_ _ _ _ _ _ _ _ _ w231 _ _ _ _ w420 _ _ _ _ _ _]
      tunnel: w18 -> [_ _ _ _ _ _ w175 _ _ _ _ w336 _ _ w412 _ _ _ _ _ _]
      tunnel: w17 -> [_ _ _ _ _ _ _ _ _ _ _ w338 _ _ w423 _ _ _ _ _ _]
      tunnel: w16 -> [_ _ _ _ _ _ _ _ _ w227 _ _ _ _ w421 _ _ _ _ _ _]
      tunnel: w15 -> [_ _ _ _ _ _ _ _ _ w226 _ _ _ _ w411 _ _ _ _ _ _]
      frame "No Match", Default {
        n10 = call "Case not matched.vi"("Case Name not Matched"=w36) -> ()
      }
      frame "Get Plot Folder" {
        # "Preserve value and restore after set-by-ref"
        # "Establish working folder in shift register before Job Directory gets overwritten by loading setup"
        n11 = Build Path(base path="Job Directory", name or relative path="gnuplots") -> (appended path=w45:path)
        n12 = local read "File Path Control"() -> (w44:path)
        n13 = case shown="False" "loadMPsetup" {
          tunnel: "setupPath" -> [w57 w65]
          tunnel: w45 -> [_ w64]
          tunnel: [w57 w62] -> w47
          tunnel: [w56 w58] -> w43
          tunnel: w44 -> [w56 w58]
          frame False {
          }
          frame True {
            # "If loadSetup requested, throw dialogue, starting in Job Directory, or last recorded setupPath"
            n14 = Empty String/Path?(string/path=w65) -> (empty?=w66:bool)
            n15 = Select(t=w64, s=w66, f=w65) -> (s? t:f=w63:path)
            n16 = control-ref of="This VI"() -> (w61:refnum<vi>)
            n17 = call "INI-FP.vi"("Mode"=enum16{"Read", "Write"}."Read", "prompt"="Select Setup to load", "VIreference"=w61, "INIfilepathIn"=w63) -> ("INIfilepathOut"=w62:path)  [unwired: 6 in, 1 out]
          }
        }
        n18 = local write "File Path Control"(w43) -> ()
        n19 = global read "Results_plotter_Global.vi" "Legend"() -> (w51:string[])
        n20 = local write "setupPath"(w47) -> ()
      }
      frame "FirstGuessPath" {
        w70 = ""
        n21 = global read "Results_plotter_Global.vi" "Current Data Filenames"() -> (w79:string)
        n22 = Array Size(array=w67) -> (size(s)=→"No of Series supplied":i32)
        n23 = case shown="True" "Set bounds using XY Plot \non Results file plotter" {
          frame False {
          }
          frame True {
            w95 = T14 {"Auto"=FALSE, "Value"=0.0} ("Min")
            n24 = call "timestampToPOSIXtime.vi"() -> ()  [unwired: 9 in, 3 out]
            n25 = local read "xAxisBounds"() -> (w105:T13)
            n26 = local read "yAxisBounds"() -> (w94:T13)
            n27 = global read "Results_plotter_Global.vi" "X plot max"() -> (w101:dbl)
            n28 = global read "Results_plotter_Global.vi" "Y plot min"() -> (w99:dbl)
            n29 = global read "Results_plotter_Global.vi" "X plot min"() -> (w100:dbl)
            n30 = global read "Results_plotter_Global.vi" "Y plot max"() -> (w98:dbl)
            n31 = Bundle By Name(cluster=w95, "Value"=w100) -> (w104:T14)
            n32 = Bundle By Name(cluster=w95, "Value"=w101) -> (w103:T14)
            n33 = Bundle By Name(cluster=w95, "Value"=w98) -> (w97:T14)
            n34 = Bundle By Name(cluster=w95, "Value"=w99) -> (w96:T14)
            n35 = Bundle By Name(cluster=w105, "Min"=w104, "Max"=w103) -> (w102:T13)
            n36 = Bundle By Name(cluster=w94, "Min"=w96, "Max"=w97) -> (w93:T13)
            n37 = local write "yAxisBounds"(w93) -> ()
            n38 = local write "xAxisBounds"(w102) -> ()
          }
        }
        n39 = call "Fast_string_Replace.vi"("Replace match with:"="_", "Input String"=w79, "matchThis"="[/]" ("regular expression")) -> ("Output String"=w82:string)  [unwired: 1 in, 1 out]
        n40 = call "Fast_string_Replace.vi"("Replace match with:"="_", "Input String"=w82, "matchThis"="__" ("regular expression")) -> ("Output String"=w80:string)  [unwired: 1 in, 1 out]
        n41 = call "Fast_string_Replace.vi"("Replace match with:"=w70, "Input String"=w80, "matchThis"=" " ("regular expression")) -> ("Output String"=w75:string)  [unwired: 1 in, 1 out]
        n42 = call "Fast_string_Replace.vi"("Replace match with:"=w70, "Input String"=w75, "matchThis"="[.]" ("regular expression")) -> ("Output String"=w72:string)  [unwired: 1 in, 1 out]
        n43 = call "Fast_string_Replace.vi"("Replace match with:"=w70, "Input String"=w72, "matchThis"=";" ("regular expression")) -> ("Output String"=w71:string)  [unwired: 1 in, 1 out]
        n44 = String Subset(string=w71, offset (0)=0, length (rest)=30 ("length (rest)")) -> (substring=w74:string)
        n45 = Build Path(base path=w89, name or relative path=w74) -> (appended path=w92:path)
      }
      frame "Sort out page title" {
        n46 = call "DistillTitle.vi"("Plot Summary in"=w118, "Show Channels with range of Values?"="Show Channels with range of Values?", "Indices to include in Page Title"="Values to include in Page Title", "String in"="") -> ("String out"=w122:string, "AvailableVariables"=w116:string[])  [unwired: 6 in]
        n47 = property on="Values to include in Page Title" class="LstBox (strict)"("Item Names"=w116) -> ()  [unwired: 2 in, 2 out]
        n48 = Concatenate Strings("Page Title Pre Block", w122, "Page Title Post Block") -> (w113:string)
        n49 = call "Fast_string_Replace.vi"("Replace match with:"=" and " ("Individual Characters to Remove"), "Input String"=w113, "matchThis"="&" ("Individual Characters to Remove")) -> ("Output String"=w110:string)  [unwired: 1 in, 1 out]
        n50 = Current VI's Path() -> (path=w128:path)
        n51 = call "Running_as_top_level.vi"("Vi path name"=w128) -> ("Top Level"=w126:bool)  [unwired: 1 out]
        n52 = call "Any_Char_Remove.vi"("Individual Characters to Remove"="{}^&", "String in"=w110) -> ("String out"=w109:string)  [unwired: 1 in]
        n53 = Build Array(w109) -> (w107:string[])
        n54 = case shown="True" w126 {
          tunnel: [w133 w136] -> w125
          tunnel: w124 -> [w133 _]
          tunnel: ["Get Filename" ("t") "Create plot directory"] -> w123
          frame False {
          }
          frame True {
            n55 = local read "File Path Control"() -> (w135:path)
            n56 = Strip Path(path=w135) -> (name=w134:string)  [unwired: 1 out]
            n57 = Build Path(base path=w135, name or relative path=w134) -> (appended path=w136:path)
          }
        }
        n58 = call "Remove_Legend3.vi"("Ordinate Strings"=w107) -> ("Array"=w108:string[])
        n59 = Index Array(array=w108) -> (element=→"Final Title":string)  [unwired: 1 in]
      }
      frame "Get Filename" {
        n60 = local read "Final Title"() -> (w145:string)
        n61 = call "Fast_string_Replace.vi"("Replace match with:"="", "Input String"=w145, "matchThis"="~" ("regular expression")) -> ("Output String"=w142:string)  [unwired: 1 in, 1 out]
        n62 = String Length(string=w142) -> (length=w147:i32)
        n63 = case shown="1, Default" w147 {
          tunnel: [w162 w163] -> w146
          tunnel: w142 -> [w162 w165]
          frame 0 {
          }
          frame 1, Default {
            n64 = Concatenate Strings(w165, "_") -> (w163:string)
          }
        }
        n65 = call "Auto_filename.vi"("Filename Max length"="Filename Max length", "Prefix"=w146) -> ("Filename"=w149:string)
        n66 = call <vilib>:"Is Name Multiplatform.vi"("filename must be valid on all platforms (F)"=TRUE ("name must work for all platforms (F)"), "filename"=w149) -> ("filename not crossplatform"=→"crossplatform problem":bool, "filename had conflict"=→"original name had conflict":bool, "suggested filename"=w141:string)  [unwired: 5 in, 2 out]
        n67 = Build Path(base path=w156, name or relative path=w141) -> (appended path=w153:path)
        n68 = Build Path(base path=w153, name or relative path=w141) -> (appended path=w160:path)
        n69 = File/Directory Info(path=w153) -> (error out=w154:errorcluster)  [unwired: 1 in, 6 out]
        n70 = Unbundle By Name(w154) -> ("status"=w152:bool)
        n71 = Select(t="Create plot directory", s=w152, f="Find a unique name") -> (s? t:f=w159:string)
      }
      frame "Find a unique name" {
        n72 = call "FindUniqueName.vi"("Max Length"=27, "PathIn"=w167) -> ("UniquedPath"=w166:path)  [unwired: 9 in]
      }
      frame "Create plot directory" {
        n73 = call "Create_directory_path.vi"("Path name"=w178) -> ("Path name Out"=w179:path)  [unwired: 2 in, 1 out]
        n74 = Strip Path(path=w178) -> (stripped path=→"File Path Control":path)  [unwired: 1 out]
        n75 = case shown="\"XY\", Default" w175 {
          tunnel: ["Sort plot points" "AddWrapforPolar"] -> w174
          frame "XY", Default {
          }
          frame "Polar" {
          }
        }
      }
      frame "Sort plot points" {
        # "Gnuplot   uses 1/1/1970 as its datum time rather than the labview value of 1/1/1904 which is 2082844800 seconds different"
        n76 = call "TimeWizard_NoSearch.vi"("Time/Date Format"="Time/Date Format", "Select Time Zone"="Select Time Zone") -> ("Format String"=→"Time Format String":string, "Formatted date/time string"=→"Formatted date/time string":string, "TZ Shift (hrs)"=→"TZ Shift (hrs)":string, "TZ Shift (sec)"=w185:dbl)  [unwired: 1 in]
        n77 = for {
          tunnel: w194 -> [w207] mode=indexing
          tunnel: [w208] -> w193 mode=indexing
          tunnel: [w200] -> w196 mode=indexing
          tunnel: w185 -> [w203]
          n78 = Unbundle(w207) -> ("Angle"=w205:dbl[], "Radius"=w206:dbl[])
          n79 = Array Max & Min(array=w205) -> (max value=w202:dbl)  [unwired: 3 out]
          n80 = call "timestampToPOSIXtime.vi"("numberToTest"=w202) -> ("subtractForPOSIX"=w201:dbl, "looksLikeTimestamp"=w200:bool)  [unwired: 8 in, 1 out]
          n81 = case shown="False" w200 {
            tunnel: w205 -> [w209 w214]
            tunnel: [w209 w213] -> w204
            tunnel: w203 -> [_ w212]
            tunnel: w201 -> [_ w210]
            frame False {
            }
            frame True {
              n82 = Subtract(x=w214, y=w210) -> (x-y=w211:dbl[])
              n83 = Add(x=w211, y=w212) -> (x+y=w213:dbl[])
            }
          }
          n84 = Bundle("Angle"=w204, "Radius"=w206) -> (w208:cluster{"Angle":dbl[], "Radius":dbl[]})  [unwired: 1 out]
        }
        n85 = Or Array Elements(Boolean array=w196) -> (logical OR=→"Time format?":bool)
      }
      frame "AddWrapforPolar" {
        n86 = for {
          tunnel: w217 -> [w225] mode=indexing
          tunnel: [w224] -> w216 mode=indexing
          tunnel: "wrapGapsUpTo:" -> [w223]
          # "Wrap plot if gap <=30deg"
          n87 = call "WrapPolarPlot.vi"("maxWrap"=w223, "thetaRin"=w225) -> ("thetaRout"=w224:cluster{"Angle":dbl[], "Radius":dbl[]})  [unwired: 9 in]
        }
      }
      frame "Save .dat file" {
        n88 = call "MakeDataFileForMultiplot.vi"("Legend"=w232, "Path"=w236, "Plot Array"=w230, "Plot Summary"=w235, "Transpose"=w231, "Error Bar Cluster"=w227, "X Axis Name"=w234, "Y Axis Name"=w233, "Error Bar Type"=w226) -> ()  [unwired: 7 in]
      }
      frame "MakePlotTitles" {
        (unwired) "-uw/U_{ref}^2__Uref (m/s)=1__LDA X (mm)=0__"
        n89 = global read "Results_plotter_Global.vi" "Ordinate Strings"() -> (w255:string[])
        n90 = global read "Results_plotter_Global.vi" "Filter 1 Strings"() -> (w248:string[])
        n91 = global read "Results_plotter_Global.vi" "Filter 2 Strings"() -> (w251:string[])
        n92 = Array Size(array=w255) -> (size(s)=w254:i32)
        n93 = call "TypesetInsideMathmode.vi"("DirtyString"=w259) -> ("Mathmode String"=→"X or theta label":string)  [unwired: 8 in, 2 out]
        n94 = call "TypesetInsideMathmode.vi"("DirtyString"=w258) -> ("Mathmode String"=→"Y or R label":string)  [unwired: 8 in, 2 out]
        n95 = call "makeNames.vi"("Strings"=w251) -> ("Names"=w250:string[])  [unwired: 10 in]
        n96 = call "makeNames.vi"("Strings"=w248) -> ("Names"=w249:string[])  [unwired: 10 in]
        n97 = Greater?(x=w254, y=1) -> (0:w252:bool)
        n98 = case shown="True" w252 {
          tunnel: w249 -> [w278 w317]
          tunnel: w250 -> [w279 w318]
          tunnel: [w275 w321] -> w245
          tunnel: [w282 w320] -> w244
          tunnel: [w283 w319] -> w247
          tunnel: w255 -> [w282 _]
          tunnel: [w273 FALSE] -> w243
          tunnel: "Swop Series and Plots" -> [w274 _]
          frame True {
            n99 = Array Size(array=w278) -> (size(s)=w281:i32)
            n100 = Array Size(array=w279) -> (size(s)=w280:i32)
            n101 = Greater?(x=w281, y=w280) -> (0:w277:bool)
            n102 = case shown="True" w277 {
              tunnel: [w291 w306] -> w283
              tunnel: w282 -> [w290 w305]
              tunnel: w279 -> [w288 w304]
              tunnel: w278 -> [w289 w302]
              tunnel: [w288 w302] -> w276
              frame False {
                n103 = Index Array(array=w289) -> (element=w292:string)  [unwired: 1 in]
                n104 = for {
                  tunnel: w292 -> [w296]
                  tunnel: w288 -> [w295]
                  tunnel: [w294] -> w291 mode=indexing
                  tunnel: w290 -> [w293] mode=indexing
                  n105 = for {
                    tunnel: w296 -> [w301]
                    tunnel: w295 -> [w300] mode=indexing
                    tunnel: [w299] -> w294 mode=indexing
                    tunnel: w293 -> [w298]
                    w297 = "__" ("string")
                    n106 = Concatenate Strings(w298, w297, w301, w297, w300, w297) -> (w299:string)
                  }
                }
              }
              frame True {
                n107 = Index Array(array=w304) -> (element=w303:string)  [unwired: 1 in]
                n108 = for {
                  tunnel: w302 -> [w310]
                  tunnel: w303 -> [w309]
                  tunnel: [w308] -> w306 mode=indexing
                  tunnel: w305 -> [w307] mode=indexing
                  n109 = for {
                    tunnel: w310 -> [w315] mode=indexing
                    tunnel: w309 -> [w314]
                    tunnel: [w313] -> w308 mode=indexing
                    tunnel: w307 -> [w312]
                    w311 = "__" ("string")
                    n110 = Concatenate Strings(w312, w311, w315, w311, w314, w311) -> (w313:string)
                  }
                }
              }
            }
            n111 = for {
              tunnel: w276 -> [w286] mode=indexing
              tunnel: [w285] -> w275 mode=indexing
              n112 = call "Fast_string_Replace.vi"("Replace match with:"="~", "Input String"=w286, "matchThis"="_" ("regular expression")) -> ("Output String"=w285:string)  [unwired: 1 in, 1 out]
            }
            n113 = Not(x=w274) -> (.not. x?=w273:bool)
          }
          frame False {
            n114 = for {
              tunnel: w317 -> [w330]
              tunnel: w318 -> [w329] mode=indexing
              tunnel: [w328] -> w319 mode=indexing
              n115 = for {
                tunnel: w330 -> [w334] mode=indexing
                tunnel: w329 -> [w333]
                tunnel: [w331] -> w328 mode=indexing
                w332 = "__" ("string")
                n116 = Concatenate Strings(w334, w332, w333, w332) -> (w331:string)
              }
            }
            n117 = for {
              tunnel: w318 -> [w327] mode=indexing
              tunnel: [w326] -> w320 mode=indexing
              # "Put space back in either side of the = sign"
              n118 = call "Edit_First_Equal.vi"("String in"=w327) -> ("String out"=w326:string)
            }
            n119 = for {
              tunnel: w317 -> [w323] mode=indexing
              tunnel: [w322] -> w321 mode=indexing
              n120 = call "Fast_string_Replace.vi"("Replace match with:"=" ", "Input String"=w323, "matchThis"="_" ("regular expression")) -> ("Output String"=w322:string)  [unwired: 1 in, 1 out]
            }
          }
        }
        "Multi_Plot" <- w243
        n121 = case shown="True" "Swop Series and Plots" {
          tunnel: w247 -> [w266 w272]
          tunnel: [w266 w271] -> w246
          tunnel: [w268 w269] -> w241
          tunnel: w245 -> [w268 w270]
          tunnel: [w267 w270] -> w239
          tunnel: w244 -> [w267 w269]
          frame False {
          }
          frame True {
            n122 = Transpose 2D Array(2D array=w272) -> (transposed array=w271:string[][])
          }
        }
        "Desired Legends" <- w246
        n123 = call "Remove_Legend3.vi"("Ordinate Strings"=w241) -> ("Array"=→"Plot Legends Auto":string[])
        n124 = call "Remove_Legend3.vi"("Ordinate Strings"=w239) -> ("Array"=→"AutoPlotTitles":string[])
      }
      frame "Gnuplot script Start" {
        n125 = local read "GraphPeripherals"() -> (w343:T17[][])
        n126 = call "setTerm.vi"("Height (in)"="Height (in)", "Width (in)"="Width (in)", "String in"="") -> ("String out"=w354:string)  [unwired: 7 in, 1 out]
        n127 = local read "Final Title"() -> (w352:string)
        n128 = call "setMultiplot.vi"("ScaleAdjust"="ScaleAdjust", "OverallTitle"=w352, "Cols"="nCols", "Rows"="nRows", "String in"=w354) -> ("nGraphs"=→"No of Graph Slots Available":i32, "String out"=w353:string)  [unwired: 4 in, 1 out]
        n129 = call "perpheralsInitialise.vi"("Legend"=w338, "PeripheralsMasterControl"="PeripheralsMasterControl", "Cols"="nCols", "Rows"="nRows", "GraphPeripheralsIn"=w343) -> ("GraphPeripheralsOut"=w344:T17[][])  [unwired: 6 in]
        n130 = local write "GraphPeripherals"(w344) -> ()
        n131 = call "setMargins.vi"("Margins"="Margins", "String in"=w353) -> ("String out"=w340:string)  [unwired: 8 in, 1 out]
        n132 = call "chainCommands.vi"("Command"="set style line 12 lc rgb '#C0C0C0' lt 1 lw 1.5 # useful pale linestyle for grids", "StringIn"=w340) -> ("StringOut"=w341:string)  [unwired: 9 in]
        n133 = Strip Path(path=w349) -> (name=w348:string)  [unwired: 1 out]
        n134 = Format Into String(format string="file=\"%s.dat\"\n" ("string"), initial string=w341, w348) -> (resulting string=w335:string)  [unwired: 1 in, 1 out]
        n135 = case shown="\"XY\", Default" w336 {
          tunnel: ["XYPlot" "PolarPlot"] -> w358
          frame "XY", Default {
          }
          frame "Polar" {
          }
        }
      }
      frame "XYPlot" {
        n136 = case shown="\"True\"" "Additional XYgnuplot" {
          selector: "Additional XYgnuplot" -> [w375 w379]
          tunnel: [w375 w378] -> w365
          frame "", Default {
          }
          frame "True" {
            n137 = Concatenate Strings("# Manual gnuplot Start" ("string"), w379, "# Manual gnuplot End" ("string")) -> (w378:string)
          }
        }
        n138 = Concatenate Strings(w367, "set border ls 12\n" ("input 2"), w365) -> (w369:string)
        "PlotCommand" <- "file index %d using 1:2 axes x1y1 title '%s' w " ("format string")
      }
      frame "PolarPlot" {
        n139 = case shown="\"True\"" "Additional Polar gnuplot" {
          selector: "Additional Polar gnuplot" -> [w404 w408]
          tunnel: [w404 w407] -> w384
          frame "", Default {
          }
          frame "True" {
            n140 = Concatenate Strings("# Manual gnuplot Start" ("string"), w408, "# Manual gnuplot End" ("string")) -> (w407:string)
          }
        }
        n141 = Select(t="set angles degrees\n", s="Angle Units", f="set angles radians\n") -> (s? t:f=w386:string)
        n142 = case shown="\"Compass\"" "AngleMode" {
          tunnel: ["90-$1" ("format string") "$1" ("format string")] -> w391
          frame "Compass" {
          }
          frame "Math", Default {
          }
        }
        n143 = Concatenate Strings(w395, w386, "set polar\nset size square\n", w384) -> (w396:string)
        n144 = case shown="\"Compass\"" "AngleMode" {
          tunnel: [90.0 0.0] -> w381
          frame "Compass" {
          }
          frame "Math", Default {
          }
        }
        n145 = Concatenate Strings("file index %d using (" ("format string"), w391, "):2 axes x1y1 title '%s' w " ("format string")) -> (w390:string)
        n146 = local read "X/Theta tics And Grids"() -> (w383:T10)
        n147 = Bundle By Name(cluster=w383, "tics.ticMin"=w381) -> (w382:T10)
        n148 = local write "PlotCommand"(w390) -> ()
        n149 = local write "X/Theta tics And Grids"(w382) -> ()
      }
      frame "Build Plot Commands" {
        n150 = local read "Desired Legends"() -> (w419:string[][])
        n151 = local read "Plot Legends Auto"() -> (w425:string[])
        n152 = Array Size(array=w419) -> (size(s)=w418:i32[])
        n153 = Index Array(array=w418) -> (element=w417:i32)  [unwired: 1 in]
        n154 = local read "AutoPlotTitles"() -> (w445:string[])
        n155 = case shown="\"Autolabel\", Default" "Y axis label" {
          tunnel: [w456 "Y or R label Manual 2"] -> w430
          frame "Autolabel", Default {
            n156 = local read "Y or R label"() -> (w456:string)
          }
          frame "Manual Label" {
          }
        }
        n157 = case shown="\"Autolabel\", Default" "X axis label" {
          tunnel: [w465 "X or theta label Manual"] -> w435
          frame "Autolabel", Default {
            n158 = local read "X or theta label"() -> (w465:string)
          }
          frame "Manual Label" {
          }
        }
        n159 = Select(t=w425, s="Plot Legends", f="Plot Legends Manual") -> (s? t:f=w424:string[])
        n160 = case shown="Default" w412 {
          tunnel: [T19 "theta" ("Axis") T19 "x" ("Axis")] -> w433
          tunnel: [T19 "r" ("Axis") T19 "y" ("Axis")] -> w432
          tunnel: ["rAxisBounds" "yAxisBounds"] -> w434
          tunnel: ["rAxisBounds" "xAxisBounds"] -> w414
          frame "Polar" {
          }
          frame Default {
          }
        }
        n161 = local read "PlotCommand"() -> (w437:string)
        n162 = global read "Results_plotter_Global.vi" "Legend"() -> (w441:string[])
        n163 = call "serialiseArray.vi"("GraphPeripherals"="GraphPeripherals") -> ("output array"=w442:T17[])  [unwired: 10 in]
        n164 = Select(t=w445, s="Individual Plot Titles", f="ManualPlotTitles") -> (s? t:f=w422:string[])
        n165 = for {
          shift-right: [w474] -> w448
          shift-left: "\n#Begin plots\n" -> [w499]
          tunnel: w424 -> [w500]
          tunnel: "Plotstyles" -> [w501]
          tunnel: w422 -> [w497] mode=indexing
          tunnel: w442 -> [w498] mode=indexing
          tunnel: w419 -> [w470] mode=indexing
          tunnel: w441 -> [w468]
          tunnel: "LegendProperties" -> [w487]
          tunnel: "Plot Title Offset (characters)" -> [w496]
          tunnel: w437 -> [w495]
          tunnel: w435 -> [w494]
          tunnel: w434 -> [w493]
          tunnel: w433 -> [w492]
          tunnel: w432 -> [w491]
          tunnel: w430 -> [w490]
          tunnel: "Y/R tics And Grids" -> [w489]
          tunnel: "X/Theta tics And Grids" -> [w488]
          tunnel: w413 -> [w472]
          tunnel: w423 -> [w486]
          tunnel: w421 -> [w482]
          tunnel: w420 -> [w481]
          tunnel: w417 -> [w480]
          tunnel: "PlotNamesNeed $$?" -> [w479]
          tunnel: "PlotTitlesNeed $$?" -> [w478]
          tunnel: w414 -> [w477]
          tunnel: w412 -> [w473]
          tunnel: w413 -> [w471]
          tunnel: w412 -> [w469]
          tunnel: w411 -> [w467]
          i -> [w485]
          # "Loops once for each graph on the multiplot"
          n166 = call "BuildPlotsOneGraph.vi"("PlotCommand"=w495, "Desired Legends"=w470, "Error Bar Type"=w467, "Plotstyles"=w501, "PlotNamesNeed $$?"=w479, "Plot Legends"=w500, "PlotArray"=w472, "Legend"=w468, "Error Bar Cluster"=w482) -> ("String out"=w475:string, "Xspan"=w483:cluster{"Max":dbl, "Min":dbl}, "Yspan"=w484:cluster{"Max":dbl, "Min":dbl})  [unwired: 4 in]
          n167 = stacked-sequence {
            seq-local: [w512 _] -> [_ w568]
            seq-local: [w508 _] -> [_ w567]
            tunnel: [_ w582] -> w476
            tunnel: w475 -> [_ w546]
            tunnel: w499 -> [_ w581]
            tunnel: w498 -> [w510 w580]
            tunnel: w497 -> [_ w573]
            tunnel: w496 -> [_ w572]
            tunnel: w494 -> [_ w559]
            tunnel: w493 -> [_ w566]
            tunnel: w492 -> [_ w571]
            tunnel: w491 -> [_ w570]
            tunnel: w490 -> [_ w563]
            tunnel: w489 -> [_ w569]
            tunnel: w488 -> [_ w552]
            tunnel: w487 -> [w511 _]
            tunnel: w486 -> [w513 _]
            tunnel: w485 -> [w507 _]
            tunnel: w484 -> [_ w564]
            tunnel: w483 -> [_ w565]
            tunnel: w481 -> [_ w558]
            tunnel: w480 -> [w506 _]
            tunnel: w478 -> [_ w556]
            tunnel: w477 -> [_ w553]
            tunnel: w471 -> [_ _]
            tunnel: w469 -> [_ w547]
            frame #0 {
              n168 = Unbundle By Name(w510) -> ("key"=w509:bool)
              n169 = case shown="\"Single Legend Below table\"" w513 {
                tunnel: [w515 w519] -> w512
                tunnel: w511 -> [w515 w520]
                tunnel: w509 -> [w514 _]
                tunnel: [w514 w518] -> w508
                tunnel: w507 -> [_ w516]
                tunnel: w506 -> [_ w517]
                frame "Legend as per array", Default {
                }
                frame "Single Legend Below table" {
                  n170 = stacked-sequence {
                    seq-local: [w522 _] -> [_ w539]
                    seq-local: [w521 _] -> [_ w538]
                    tunnel: w520 -> [_ w545]
                    tunnel: w516 -> [_ w542]
                    tunnel: [_ w541] -> w519
                    tunnel: [_ w540] -> w518
                    tunnel: w517 -> [w524 _]
                    frame #0 {
                      n171 = local read "No of Graph Slots Available"() -> (w525:i32)
                      n172 = Greater?(x=w525, y=w524) -> (0:w523:bool)
                      n173 = case shown="True" w523 {
                        tunnel: [0.6 ("\"At\" location.Xvalue") w532] -> w522
                        tunnel: [-0.03 ("\"At\" location.Yvalue") w529] -> w521
                        frame False {
                        }
                        frame True {
                          n174 = local read "nCols"() -> (w536:u8)
                          n175 = local read "nRows"() -> (w530:u8)
                          n176 = Decrement(x=w536) -> (x-1=w537:u8)
                          n177 = Increment(x=w530) -> (x+1=w528:u8)
                          n178 = Divide(x=w537, y=w536) -> (x/y=w533:dbl)
                          n179 = Divide(x=1.0, y=w528) -> (x/y=w529:dbl)
                          n180 = Divide(x=0.7, y=w536) -> (x/y=w534:dbl)
                          n181 = Add(x=w533, y=w534) -> (x+y=w532:dbl)
                        }
                      }
                    }
                    frame #1 {
                      w543 = "screen" ("\"At\" location.XcoordSys")
                      # "Use \"screen\" coordinates to place legend at bottom-center\nof entire \"screen\" of graphs; update legend cluster to \nreflect this."
                      # "Only legend the first graph"
                      n182 = Equal To 0?(x=w542) -> (x = 0?=w540:bool)
                      n183 = Bundle By Name(cluster=w545, "Location"="at", "\"At\" location.XcoordSys"=w543, "\"At\" location.Xvalue"=w539, "\"At\" location.YcoordSys"=w543, "\"At\" location.Yvalue"=w538) -> (w541:T6)
                      n184 = local write "LegendProperties"(w541) -> ()
                    }
                  }
                }
              }
            }
            frame #1 {
              n185 = local read "Multi_Plot"() -> (w561:bool)
              n186 = case shown="False" w558 {
                tunnel: w563 -> [w589 w598]
                tunnel: [w589 w597] -> w562
                tunnel: w561 -> [w592 w595]
                tunnel: [w590 w594] -> w560
                tunnel: w559 -> [w591 w594]
                frame True {
                  n187 = Select(t="", s=w592, f=w591) -> (s? t:f=w590:string)
                }
                frame False {
                  n188 = Select(t="", s=w595, f=w598) -> (s? t:f=w597:string)
                }
              }
              n189 = Unbundle By Name(w580) -> ("title"=w579:bool, "Xtic"=w577:bool, "Xlab"=w576:bool, "Ytic"=w575:bool, "Ylab"=w574:bool)
              n190 = call "TypesetInsideMathmode.vi"("Needs $$?"=w556, "DirtyString"=w573) -> ("ChosenStringtype"=w557:string)  [unwired: 7 in, 2 out]
              n191 = call "setTitle.vi"("Offset"=w572, "Set?"=w579, "Title"=w557, "String in"=w581) -> ("String out"=w578:string)  [unwired: 6 in, 1 out]
              n192 = local read "Time Format String"() -> (w554:string)
              n193 = local read "Time format?"() -> (w555:bool)
              n194 = call "setKey.vi"("LegendProperties"=w568, "Set?"=w567, "String in"=w578) -> ("String out"=w551:string)  [unwired: 7 in, 1 out]
              n195 = call "AxisControl.vi"("String in"=w551, "AxisBounds"=w566, "ticsAndGrids"=w569, "Axis"=w570, "ShowNumbers?"=w575, "ShowLabel?"=w574, "Axis Label"=w562, "DataSpan"=w564) -> ("String out"=w549:string)  [unwired: 6 in, 1 out]
              n196 = case shown="\"Polar\"" w547 {
                tunnel: w549 -> [w583 w585]
                tunnel: [w583 w584] -> w548
                tunnel: w546 -> [_ w586]
                frame "XY", Default {
                }
                frame "Polar" {
                  n197 = Concatenate Strings(w585, "set table \"outfile.txt\"\n" ("string"), w586, "rmax = GPVAL_R_MAX\nrmin = GPVAL_R_MIN\nunset table\n" ("string")) -> (w584:string)
                }
              }
              n198 = call "AxisControl.vi"("String in"=w548, "AxisBounds"=w553, "Time Format String"=w554, "ticsAndGrids"=w552, "Axis"=w571, "Time format?"=w555, "ShowNumbers?"=w577, "ShowLabel?"=w576, "Axis Label"=w560, "DataSpan"=w565) -> ("String out"=w550:string)  [unwired: 4 in, 1 out]
              n199 = Concatenate Strings(w550, w546) -> (w582:string)
            }
          }
          n200 = case shown="\"Polar\"" w473 {
            tunnel: w476 -> [w502 w505]
            tunnel: [w502 w504] -> w474
            frame "XY", Default {
            }
            frame "Polar" {
              n201 = Concatenate Strings(w505, "unset label\n" ("string")) -> (w504:string)
            }
          }
        }
        n202 = Concatenate Strings(w447, w448, "\nunset multiplot\n") -> (w453:string)
      }
      frame "Write gnuplot file" {
        w606 = FALSE  # append to file? (new file:F)
        w607 = FALSE  # advisory dialog? (display:T)
        n203 = Strip Path(path=w603) -> (stripped path=w600:path)  [unwired: 1 out]
        n204 = Build Path(base path=w600, name or relative path="gnuplot_script.txt") -> (appended path=w608:path)
        n205 = call "Write_Characters_To_File.vi"("file path (dialog if empty)"=w608, "advisory dialog? (display:T)"=w607, "character string"=w599, "append to file? (new file:F)"=w606) -> ()  [unwired: 1 in, 4 out]
      }
      frame "Execute shell script" {
        n206 = call "Run_Gnuplot_Script.vi"("logfileName"=w610, "targetFile"=w611) -> ()  [unwired: 1 in]
      }
      frame "Has pdf been generated?" {
        n207 = Current VI's Path() -> (path=w617:path)
        n208 = call "Running_as_top_level.vi"("Vi path name"=w617) -> ("Top Level"=w618:bool)  [unwired: 1 out]
        n209 = call "Create_copy_of_pdf in day folder.vi"("Top Level"=w618, "Path name Out"=w619) -> ()  [unwired: 1 in]
        n210 = Select(t="Open Standard output file" ("f"), s="OpenLogfile?", f="End") -> (s? t:f=w620:string)
        n211 = Select(t="Show Re-Run Gnuplot?", s="Show Script Editor?", f=w620) -> (s? t:f=w624:string)
      }
      frame "Show Re-Run Gnuplot?" {
        n212 = Strip Path(path=w632) -> (stripped path=w631:path)  [unwired: 1 out]
        n213 = call "Re_run_Gnuplot.vi"("Plot folder (dialog if empty)"=w631) -> ()  [unwired: 1 in, 3 out]
      }
      frame "Open Standard output file" {
        n214 = Strip Path(path=w642) -> (stripped path=w639:path)  [unwired: 1 out]
        n215 = Format Into String(format string="open \"%s\"", w640) -> (resulting string=w638:string)  [unwired: 2 in, 1 out]
        n216 = call <vilib>:"System Exec.vi"("working directory"=w639, "command line"=w638) -> ()  [unwired: 4 in, 6 out]
      }
      frame "End" {
        w649 = enum16{"Read", "Write"}."Write" ("Mode")
        # "Save to user-named file only on request"
        # "Always auto-save setup"
        n217 = call "replaceFileExtension.vi"("replacementExtension"="-setup.ini", "pathIn"=w648) -> ("pathOut"=w651:path)  [unwired: 8 in, 1 out]
        n218 = control-ref of="This VI"() -> (w650:refnum<vi>)
        n219 = case shown="True" "saveMPsetup" {
          tunnel: w650 -> [_ w664]
          tunnel: w649 -> [_ w663]
          tunnel: w648 -> [_ w662]
          frame False {
          }
          frame True {
            n220 = Strip Path(path=w662) -> (stripped path=w661:path)  [unwired: 1 out]
            n221 = call "INI-FP.vi"("Mode"=w663, "prompt"="Where to save Multiplot setup?", "VIreference"=w664, "INIfilepathIn"=w661) -> ()  [unwired: 6 in, 2 out]
          }
        }
        n222 = call "INI-FP.vi"("Mode"=w649, "prompt"="", "VIreference"=w650, "INIfilepathIn"=w651) -> ()  [unwired: 6 in, 2 out]
        n223 = global write "Results_plotter_Global.vi" "New Chs In"(string[] [] ("New Chs In")) -> ()
      }
    }
    "gnuplotScript" <- w20
  }
  "AuditTrail" <- w6
  "Saved Automatically?" <- FALSE
